vi "Control Experiment SM.vi"() -> ()   [LabVIEW 2016, in "Control Experiment SM.lvclass"]
doc: "Use this VI to help configure your experiment.\n1. Choose Pickering or Not Pickering\n2. Configure the Electrode control to show which electrode is connected to which lockin\n3. Choose a Label for each electrode to configure Krohn Hite amplifier automatically\n4. Easily set all Krohn Hite channels to be \"all ground\" or \"all differential\" mode\n5. Fill out information about you and your device in the lower left corner\n6. When you are finished, or when you want to update the amplifiers, click the \"CREATE OUTPUT\" button located in upper right. Clicking this button will set the amplifiers, Pickering switch (if you have one), and write information to a functional global variable that you can easily read from elsewhere in your program"
uses:
  Control Experiment SM.lvclass
  Typedefs/Instrument--enum.ctl
  <userlib>/LevyLab/Krohn Hite 7008/typedefs/Shunt-Enum.ctl
  <userlib>/LevyLab/Krohn Hite 7008/Instrument.KH7008.lvclass
  <userlib>/LevyLab/Levylab Instruments/SMOs/Configuration/Configuration.lvclass
  <userlib>/LevyLab/Lockin-Multichannel/Instrument.Lockin/Instrument.Lockin.lvclass
  <userlib>/LevyLab/Levylab Instruments/Instrument Types/Cryostat/Instrument.Cryostat.lvclass
  <userlib>/LevyLab/Levylab Instruments/Instrument Types/CBridge/Instrument.CBridge.lvclass
  <userlib>/LevyLab/Levylab Instruments/Instrument Types/Optical Delay Line/Instrument.OpticalDelayLine.lvclass
  <userlib>/LevyLab/Levylab Instruments/Instrument Types/Strain/Instrument.Strain.lvclass
  <userlib>/LevyLab/Levylab Instruments/Instrument Types/VNA/Instrument.VNA.lvclass
  <userlib>/LevyLab/Levylab Instruments/Instrument Types/VSource/Instrument.VSource.lvclass
  Typedefs/KH Mode-enum.ctl
  <userlib>/LevyLab/Krohn Hite 7008/typedefs/Input Configuration-Enum.ctl
  <userlib>/LevyLab/Krohn Hite 7008/typedefs/Gain-Enum.ctl
  <userlib>/LevyLab/Krohn Hite 7008/typedefs/SetAll-Array.ctl
  <userlib>/LevyLab/Krohn Hite 7008/typedefs/SetAll-Cluster.ctl
  <userlib>/LevyLab/Krohn Hite 7008/typedefs/Channel-Enum.ctl
  <userlib>/LevyLab/Krohn Hite 7008/typedefs/Filter-Enum.ctl
  <userlib>/LevyLab/Krohn Hite 7008/typedefs/Coupling-Enum.ctl
  <vilib>/addons/_JKI.lib/REST Client/classes/REST Client/HTTP Header.ctl
  Typedefs/UI Controls --cluster.ctl
  <userlib>/LevyLab/Levylab Instruments/SMOs/Logger.PGSQL/Logger.PGSQL.lvclass
  C:/Program Files (x86)/National Instruments/LabVIEW 2016/vi.lib/JKI/JKI SMO/SMO/SMO.lvclass
  Control Experiment SM.lvclass/Control Experiment SM.ctl
  <vilib>/Utility/sysdir.llb/System Directory Type.ctl
  <userlib>/_MGI/File/MGI Create Directory Chain Behavior Enum.ctl
  Typedefs/Control Experiment JSON--cluster.ctl
  <userlib>/LevyLab/Krohn Hite 7008/Instrument.KH7008.lvclass/Instrument.KH7008.ctl
  <userlib>/_OpenG.lib/file/file.llb/File Exists - Scalar__ogtk.vi
  <vilib>/Platform/browser.llb/Open URL in Default Browser (string).vi
  <userlib>/_OpenG.lib/array/array.llb/Remove Duplicates from 1D Array (Variant)__ogtk.vi
  <vilib>/addons/_JKI.lib/Serialization/JSON/JKI JSON Serialization.lvlib
  <vilib>/addons/_JKI.lib/REST Client/classes/REST Client/REST Client.lvclass
  <vilib>/JKI/JKI SMO/SMO/SMO.lvclass
panel:
  in  "I'm Finished Taking Data!":bool
  out "Values have changed":bool
  in  "Create Output":bool
  in  "OK":bool
  out "Control Experiment":refnum<class "Control Experiment SM.lvclass">
  in  "C.E.":refnum<class "Control Experiment SM.lvclass">
  in  "Tab Control":T1(tab)
  in  "DC Coupled":bool=TRUE
  in  "Bandwidth Filter":bool=TRUE
  in  "#AO":u32=8
  in  "Gain":dbl[](array[numeric])=[1.0, 1.0, 1.0, 1.0, 1.0, 1.0, 1.0, 1.0]
  in  "KH":T5={"KH #"=[0, 1, 2, 3, 4, 5, 6, 7], "KH Configuration"=[enum."Differential", enum."Differential", enum."SE+ (-gnd)", enum."SE+ (-gnd)", enum."Ground", enum."Differential", enum."Ground", enum."Differential"], "KH Gain"=[enum."1x", enum."1000x", enum."1x", enum."10x", enum."1x", enum."1x", enum."1x", enum."1x"], "KH Shunt Resistor"=[enum."50k Ohms", enum."50k Ohms", enum."Open", enum."Open", enum."Open", enum."50k Ohms", enum."Open", enum."Open"]}
  in  "Lockin":T7={"AI"=[1, 2, 3, 4, 5, 6, 7, 8], "Electrode"=["1", "2", "4", "3", "", "26", "", ""], "Label"=[2, 14, 3, 4, 0, 1, 0, 0], "Electrode Config"=[enum."Current", enum."Gate", enum."Voltage (SE)", enum."Voltage (SE)", enum."Ground", enum."Current", enum."Ground", enum."Voltage (Diff)"]} {"Label" items=["", "I+", "I-", "V1+", "V1-", "V2+", "V2-", "V3+", "V3-", "V4+", "V4-", "dV1", "dV2", "dV3", "Vsg", "Vbg"]}
  in  "#AI":u32=8
  in  "KH All Buttons":T8(radio)
  in  "Defualt Shunt Resistor":T4=enum."50k Ohms"
  in  "Description":string="this is a test"
  in  "Sample (SAXXXX)":string="TEST"
  in  "Device (YYYYMMDD)":string="20200113"
  in  "Instrument":T9
  in  "Username":string="Patrick"
  in  "non KH":T10={"AO"=[], "Electrodes 2"=["27"], "Labels 2"=[1], "unused"=[]} {"Labels 2" items=["", "I+", "I-", "V1+", "V1-", "V2+", "V2-", "V3+", "V3-", "V4+", "V4-", "dV1", "dV2", "dV3", "Vsg", "Vbg"]}
  in  "Strain Cell Address":refnum<visa-resource-name>="GPIB0::INSTR38"
  in  "Capacitance Bridge Address":refnum<visa-resource-name>
  in  "C Bridge?":bool=TRUE
  in  "Strain Cell?":bool=TRUE
  in  "Krohn Hite?":bool=TRUE
  in  "KH Addresses":refnum<visa-resource-name>[](array[refnum])=["COM1"] caption="KH Address[A,B,C,...]"
  in  "Lockin Address":string
  in  "Ring":u16(ring) items=["----Sweep Control----", "Sweep Control.vi", "Continuous B Sweep.vi", "----Transport----", "IV.vi", "IV_Sweep.vi", "Lockin_time.vi", "Lockin_Vsg.vi", "Lockin_sweep.vi", "Lockin_AIWFM_time.vi", "THz_TimeDelay.vi", "Sweep_AIWFM_time.vi"]
  in  "Open VI":bool
  in  "Open Lockin":bool
  in  "Write Pickering Config":bool
  in  "Read Pickering Config":bool
  in  "AWS Credentials":path=path "G:/My Drive/ansom/Data" caption="AWS Credentials (File with AWS access key and secret access key"
  out "Refresh Token Out":string="0/0ccae0b202a2d5ce21e5be9cd72246b8"
  in  "Default Path":path=path "G:/My Drive/ansom/Data" caption="Default Path (Do not add your instrument name here)(Typ. G:\\My Drive\\ansom\\Data)"
  out "Comments":string="Device: \r  Device Name: TEST.20200113\r  Computer: ASTARTES\r  User: Patrick\r  Instrument: AGILENT\r  Description: |\r    this is a test\r\rExperiment: \r  Time: 2020-02-25T09:02:18\r  Description: |\r\rSweep: \r- Loop1: [OFF, 0.000000]\r- Loop2: [OFF, 0.000000]\r- Loop3: [OFF, 0.000000]\r- Loop4: [OFF, 0.000000]\r\rWiring: \r- Electrode 27: Lockin 1, I+, KH1 Channel 1, Differential, 1x, 50k Ohms\r\rLockin: \r  AO: \r  \r  REF: \r  \r  Sampling: \r  - Fs: \r  - N: \r"
  out "Device Folder":path=path "G:/My Drive/ansom/Data/AGILENT/TEST.20200113" caption="(\\base path\\project\\device\\ )"
  out "JSON String":string="{\r\n    \"Device\":{\r\n        \"Device\":\"TEST.20200113\",\r\n        \"User\":\"Patrick\",\r\n        \"Time\":\"2020-02-25T09:02:24\",\r\n        \"Computer Name\":\"ASTARTES\"\r\n    },\r\n    \"Wiring\":{\r\n        \"Lockin Ch\":[\r\n            1,\r\n            2,\r\n            3,\r\n            4,\r\n            5,\r\n            6,\r\n            7,\r\n            8\r\n        ],\r\n        \"KH Electrodes\":[\r\n            \"27\"\r\n        ],\r\n        \"KH Labels\":[\r\n            \"I+\"\r\n        ],\r\n        \"Other Electrodes\":[\r\n            \"27\"\r\n        ],\r\n        \"Other Labels\":[\r\n            \"I+\"\r\n        ]\r\n    }\r\n}"
  in  "Labels Strings":string[](array[string])=["", "I+", "I-", "V1+", "V1-", "V2+", "V2-", "V3+", "V3-", "V4+", "V4-", "dV1", "dV2", "dV3", "Vsg", "Vbg"]
  out "YAML example":string="description: This is a dummy dataset which mimics smFRET data.\n\nsetup:\n    ## Mandatory fields\n    num_pixels: 2                # using 2 detectors\n    num_spots: 1                 # a single confocal excitation\n    num_spectral_ch: 2           # donor and acceptor detection\n    num_polarization_ch: 1       # no polarization selection\n    num_split_ch: 1              # no beam splitter\n    modulated_excitation: False  # CW excitation, no modulation\n    lifetime: False              # no TCSPC in detection\n\n    ## Optional fields\n    excitation_wavelengths:      # List of excitation wavelenghts\n       - !!float 532e-9\n    excitation_cw:               # List of booleans, True if wavelength is CW\n       - True\n    detection_wavelengths:       # Nominal center wavelength for each for detection ch\n       - !!float 580e-9\n       - !!float 640e-9\n\nsample:\n  sample_name: describe the sample here\n  buffer_name: describe the buffer here\n  dye_names: 'Cy3B, ATTO647N'   # Comma separates names of fluorophores\n\nidentity:\n    author: Author Name\n    author_affiliation: Name of Research Institution\n\nprovenance:\n    filename: 'photon_data.hdf5'\n    software: Acquisition Software Name\n\nphoton_data:\n    timestamps_specs:\n        timestamps_unit: !!float 10e-9  # 10 ns\n    measurement_specs:\n        measurement_type: smFRET\n        detectors_specs:\n            spectral_ch1: [0]  # list of donor's detector IDs\n            spectral_ch2: [1]  # list of acceptor's detector IDs"
  in  "String":string
  # "SANDBOX:"
  # "Sample"
  # "Krohn Hite"
  # "Lockin"
  # "Lockin"
  # "Krohn Hite"
  # "Other"
  # "Device and Project Description"
  # "Hardware Configuration"
  # "Experiment VIs"
  # "Lockin (Local)"
  # "Path Configuration"
  # "Use this VI to help configure your experiment.\n1. Choose Pickering or Not Pickering\n2. Configure the Electrode control to show which electrode is connected to which lockin\n3. Choose a Label for each electrode to configure Krohn Hite amplifier automatically\n4. Easily set all Krohn Hite channels to be \"all ground\" or \"all differential\" mode\n5. Fill out information about you and your device in the lower left corner\n6. When you are finished, or when you want to update the amplifiers, click the \"CREATE OUTPUT\" button located in upper right.\nClicking this button will set the amplifiers, Pickering switch (if you have one), and write information to a functional global variable that you can easily read from elsewhere in your program"
  # "If you want to have new labels for the \"Labels\" field you can type them here"
  # "The magic words are:\nI\nVsg\nVbg\ndV\nV"
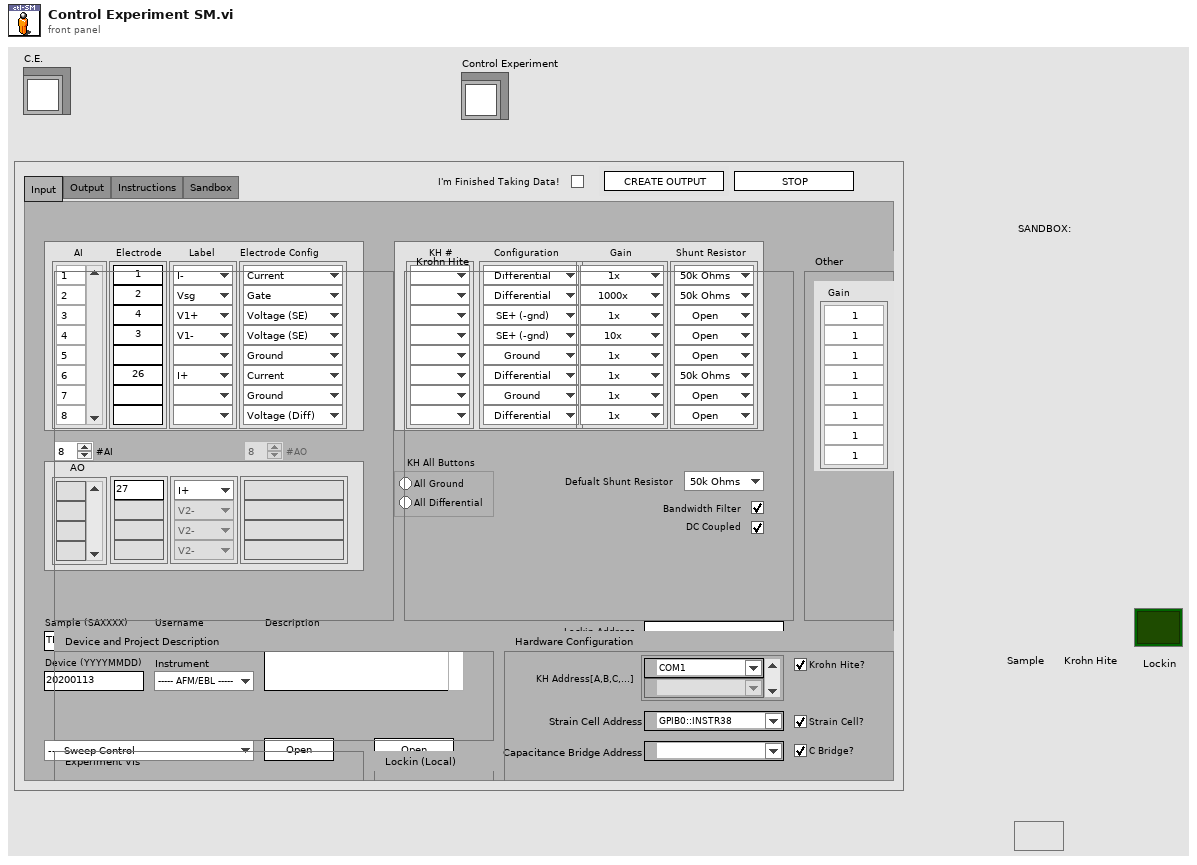
[diagram p1: front panel]
types:
  T1 = enum32{"Input", "Pickering", "Output", "Instructions", "Sandbox"}
  T2 = typedef "Instrument.KH7008.lvclass/Input Configuration-Enum.ctl" = enum16{"Ground", "SE+ (-gnd)", "SE- (+gnd)", "Differential"}
  T3 = typedef "Instrument.KH7008.lvclass/Gain-Enum.ctl" = enum16{"1x", "10x", "100x", "1000x"}
  T4 = typedef "Instrument.KH7008.lvclass/Shunt-Enum.ctl" = enum16{"Open", "50 Ohms", "500 Ohms", "5k Ohms", "50k Ohms", "10M Ohm"}
  T5 = cluster{"KH #":u16[], "KH Configuration":T2[], "KH Gain":T3[], "KH Shunt Resistor":T4[]}
  T6 = typedef "Control Experiment SM.lvclass/KH Mode-enum.ctl" = enum16{"Ground", "Current", "Voltage (SE)", "Voltage (Diff)", "Gate"}
  T7 = cluster{"AI":u32[], "Electrode":string[], "Label":u16[], "Electrode Config":T6[]}
  T8 = enum32{"No Selection", "All Ground", "All Differential"}
  T9 = typedef "Control Experiment SM.lvclass/Instrument--enum.ctl" = enum16{"----- AFM/EBL -----", "AGILENT", "CYPHER", "Gemini2", "JEOL", "MFP3D", "----- Cryostat -----", "CF900", "DR200", "MNK", "PPMS 1", "PPMS 2", "PPMS 3", "----- Optics -----", "THz 1", "THz 2"}
  T10 = cluster{"AO":string[], "Electrodes 2":string[], "Labels 2":u16[], "unused":string[]}
  T11 = enum16{"A 1", "A 2", "A 3", "A 4", "A 5", "A 6", "A 7", "A 8", "B 1", "B 2", "B 3", "B 4", "B 5", "B 6", "B 7", "B 8", "none"}
  T12 = enum32{"invalid app kind", "Development System", "Run Time System", "Student Edition", "Embedded LabVIEW", "Evaluation", "Custom"}
  T13 = enum32{"Invalid", "Standard", "Closed", "Hidden", "Minimized", "Maximized"}
  T14 = typedef "MGI Create Directory Chain Behavior Enum.ctl" = enum16{"Auto Detect", "Path Contains a File", "Path Does Not Contain a File"}
  T15 = typedef "Instrument.KH7008.lvclass/SetAll-Cluster.ctl" = cluster{"Channel":T16, "Gain":T3, "Bandwidth Filter":T17, "Shunt Resistor":T4, "Coupling":T18, "Input Config":T2}
  T16 = typedef "Instrument.KH7008.lvclass/Channel-Enum.ctl" = enum16{"Channel 1", "Channel 2", "Channel 3", "Channel 4", "Channel 5", "Channel 6", "Channel 7", "Channel 8"}
  T17 = typedef "Instrument.KH7008.lvclass/Filter-Enum.ctl" = enum16{"OFF", "ON"}
  T18 = typedef "Instrument.KH7008.lvclass/Coupling-Enum.ctl" = enum16{"AC", "DC"}
  T19 = enum16{"GSR", "Research Projects", "Undergrads", "Researchers", "Hardware", "Software", "LevyLab", "Samples", "Manuscripts", "AoT", "WorkStudy"}
  T20 = enum16{"A 1", "A 2", "A 3", "A 4", "A 5", "A 6", "A 7", "A 8", "B 1", "B 2", "B 3", "B 4", "B 5", "B 6", "B 7", "B 8", "none"}[]
  T21 = typedef "Control Experiment SM.lvclass/Experiment Description--cluster.ctl" = cluster{"User":string, "Device":string, "Device Path":path, "Device Description":string, "Experiment Path":path, "Experiment Description":string, "Instrument":T9, "Sweep":cluster{"key":string, "value":variant}[], "Device Description JSON":string, "Experiment Description JSON":string}
  T22 = typedef "Control Experiment SM.lvclass/Wiring Description--cluster.ctl" = cluster{"Lockin Ch":i32[], "KH":cluster{"Electrodes":string[], "Labels":string[]}, "not KH":cluster{"Electrodes":string[], "Labels":string[]}}
  T23 = typedef "Instrument.KH7008.lvclass/SetAll-Array.ctl" = T15[]
  T24 = typedef "Control Experiment SM.lvclass/UI Controls --cluster.ctl" = cluster{"Sample":string, "Device":string, "Username":string, "Description":string, "Default Path":path, "AWS Path":path, "Instrument":T9, "Lockin?":bool, "Lockin Address":string, "Krohn Hite?":bool, "KH Addresses":refnum<visa-resource-name>[], "KH All Buttons":enum32{"No Selection", "All Ground", "All Differential"}, "Strain Cell?":bool, "Strain Cell Address":refnum<visa-resource-name>, "C Bridge?":bool, "Capacitance Bridge Address":refnum<visa-resource-name>, "Lockin":cluster{"AI":u32[], "Electrode":string[], "Label":u16[], "Electrode Config":T6[]}, "KH":cluster{"KH #":enum16{"A 1", "A 2", "A 3", "A 4", "A 5", "A 6", "A 7", "A 8", "B 1", "B 2", "B 3", "B 4", "B 5", "B 6", "B 7", "B 8", "none"}[], "KH Configuration":T2[], "KH Gain":T3[], "KH Shunt Resistor":T4[], "Filter":bool, "DC Coupled":bool}, "non KH":cluster{"Scroll Bar":string[], "Electrodes 2":string[], "Labels 2":u16[], "unused":string[]}, "#AI":u32}
  T25 = typedef "REST Client.lvlib/REST Client.lvclass/HTTP Header.ctl" = cluster{"header":string, "value":string}
  T26 = cluster{"Core":cluster{"Current VI Reference":refnum<vi>, "Close Panel on Exit?":bool}, "C.E.":refnum<class "Control Experiment SM.lvclass">, "Experiment":T21, "Wiring Configuration":T22, "Channel Settings":cluster{"Channel Setting":T23}[], "KH All Buttons":enum32{"No Selection", "All Ground", "All Differential"}, "Lockin":cluster{"AI":u32[], "Electrode":string[], "Label":u16[], "Electrode Config":T6[]}, "KH":cluster{"KH #":u16[], "KH Configuration":T2[], "KH Gain":T3[], "KH Shunt Resistor":T4[]}, "non KH":cluster{"AO":string[], "Electrodes 2":string[], "Labels 2":u16[], "unused":string[]}, "UI":T24, "Asana":cluster{"Authentication Info":cluster{"Client ID":string, "Client Secret":string, "Redirect URI":string, "Token Endpoint":string, "Scope":string}, "Authentication Header":T25[], "Refresh Token":string, "Time Stamp":timestamp}, "Logger":refnum<class "Logger.PGSQL.lvclass">, "Config":refnum<class "Configuration.lvclass">, "VI paths":path[]}
  T27 = cluster{"Authentication Info":cluster{"Client ID":string, "Client Secret":string, "Redirect URI":string, "Token Endpoint":string, "Scope":string}, "Authentication Header":T25[], "Refresh Token":string, "Time Stamp":timestamp}
  T28 = cluster{"Current VI Reference":refnum<vi>, "Close Panel on Exit?":bool}
  T29 = typedef "System Directory Type.ctl" = i32
  T30 = cluster{"Scroll Bar":string[], "Electrodes 2":string[], "Labels 2":u16[], "unused":string[]}
  T31 = typedef "Control Experiment SM.lvclass/Control Experiment JSON--cluster.ctl" = cluster{"Device":cluster{"Device":string, "User":string, "Time":string, "Computer Name":string}, "Wiring":cluster{"Lockin Ch":u32[], "KH Electrodes":string[], "KH Labels":string[], "Other Electrodes":string[], "Other Labels":string[]}}
  T32 = cluster{"Client ID":string, "Client Secret":string, "Redirect URI":string, "Token Endpoint":string, "Scope":string}
  T33 = cluster{"gid":string, "name":string, "resource_type":string}[]
  T34 = cluster{"id":i64, "gid":string, "resource_type":string, "name":string}[]
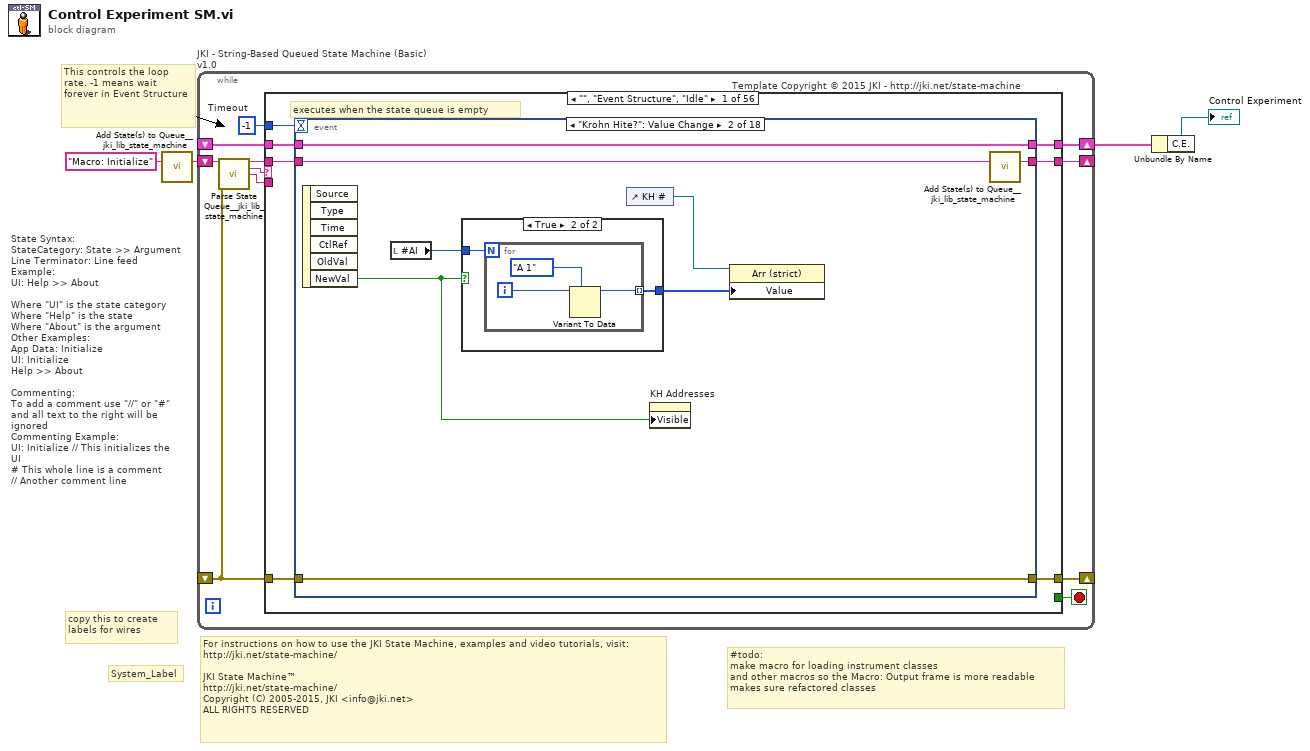
[diagram p0: block diagram]
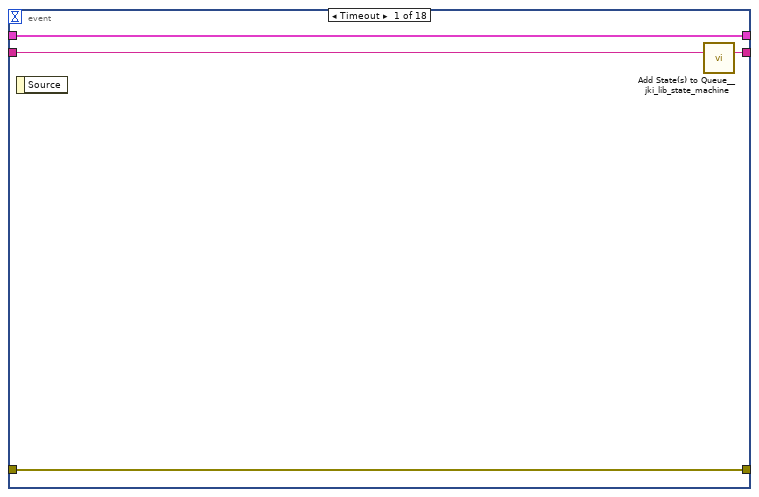
[diagram p2: hidden frame]
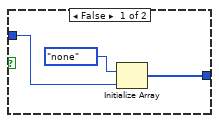
[diagram p3: hidden frame]
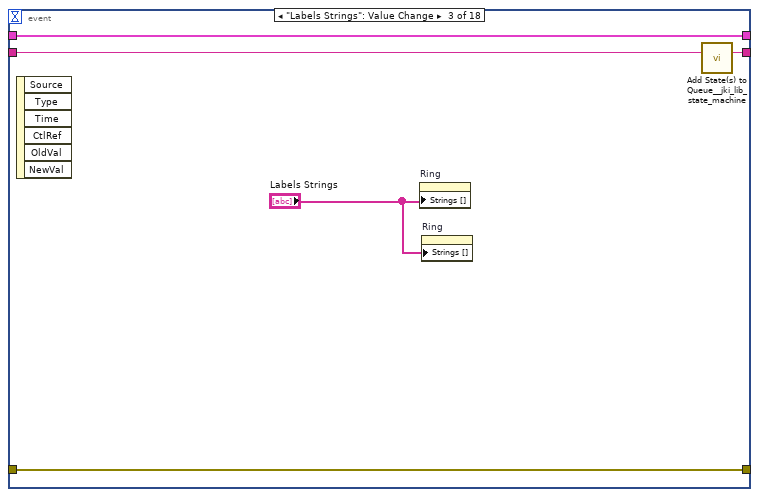
[diagram p4: hidden frame]
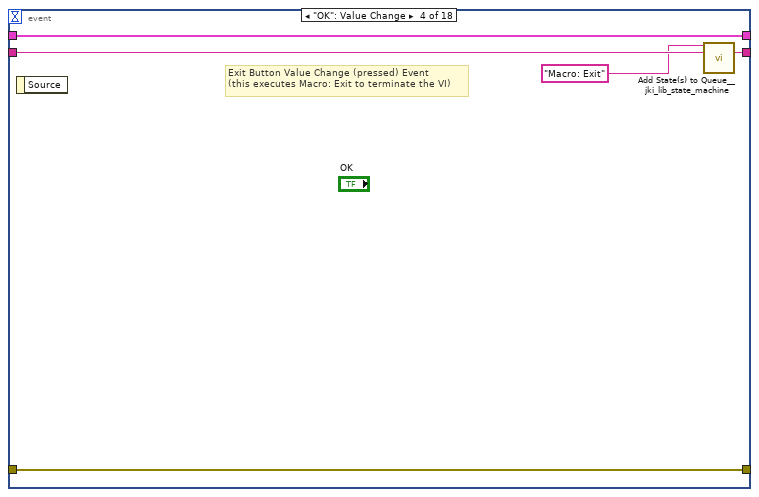
[diagram p5: hidden frame]
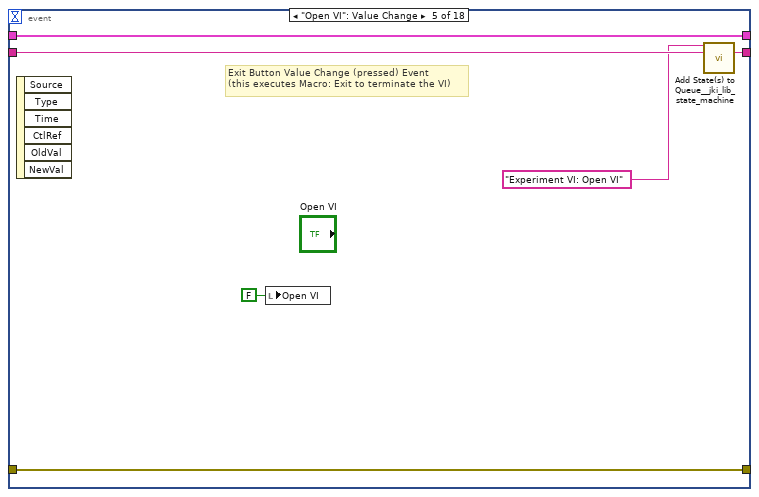
[diagram p6: hidden frame]
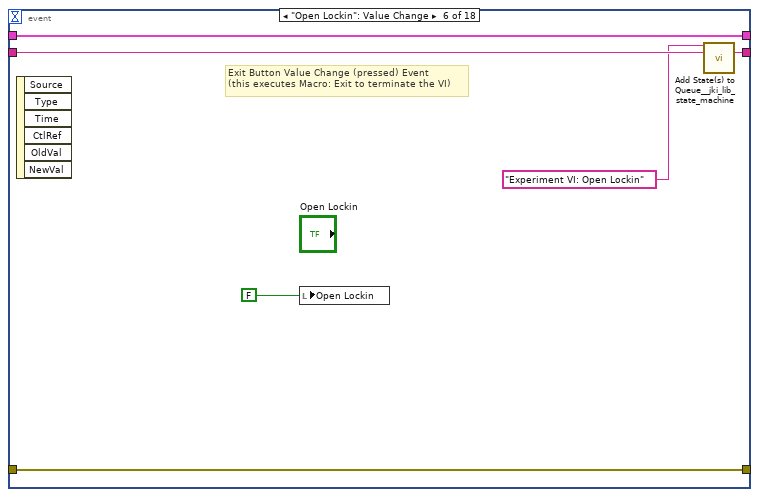
[diagram p7: hidden frame]
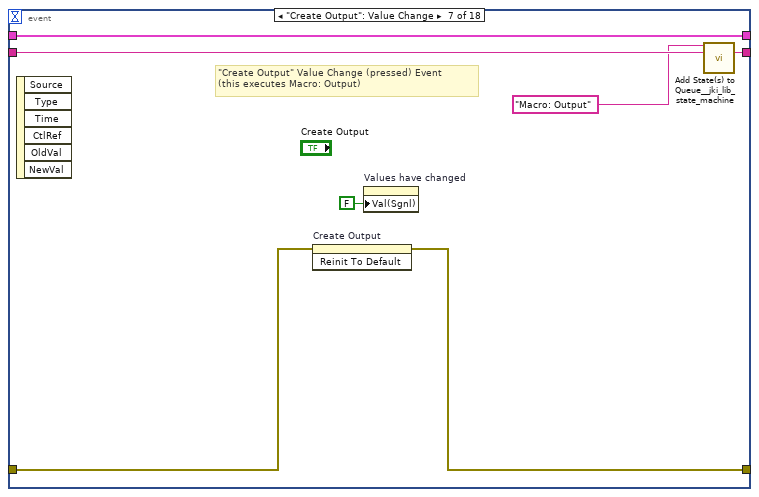
[diagram p8: hidden frame]
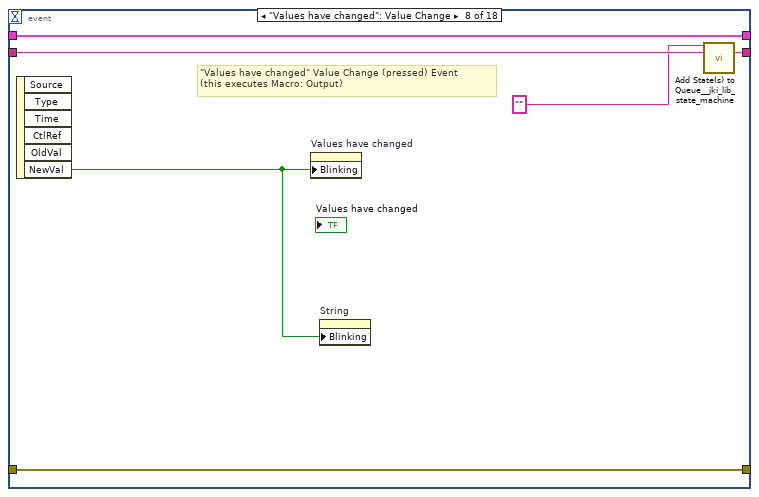
[diagram p9: hidden frame]
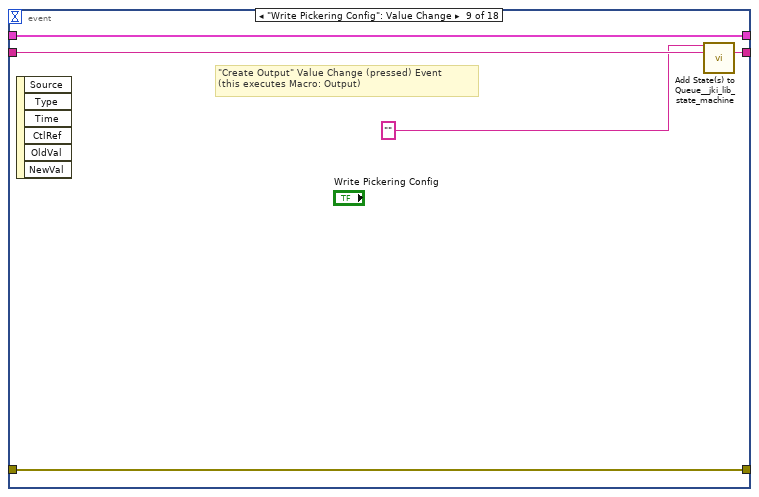
[diagram p10: hidden frame]
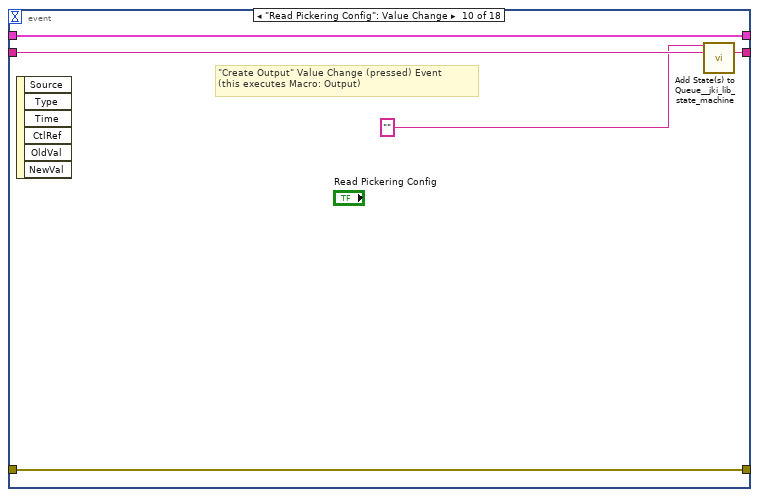
[diagram p11: hidden frame]
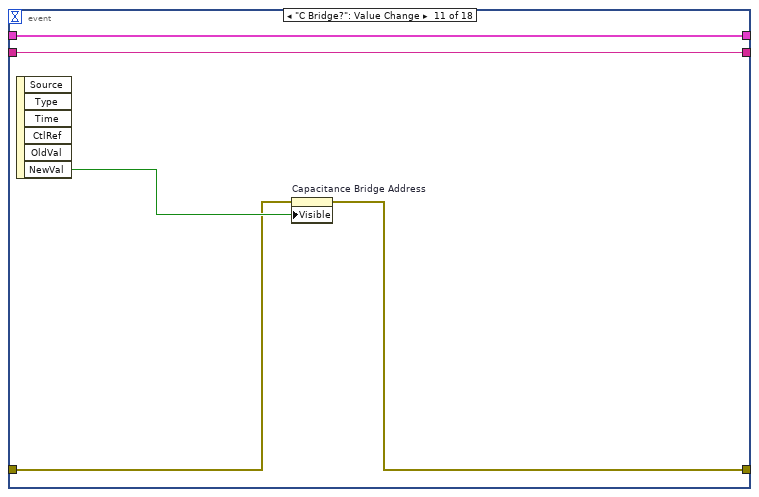
[diagram p12: hidden frame]
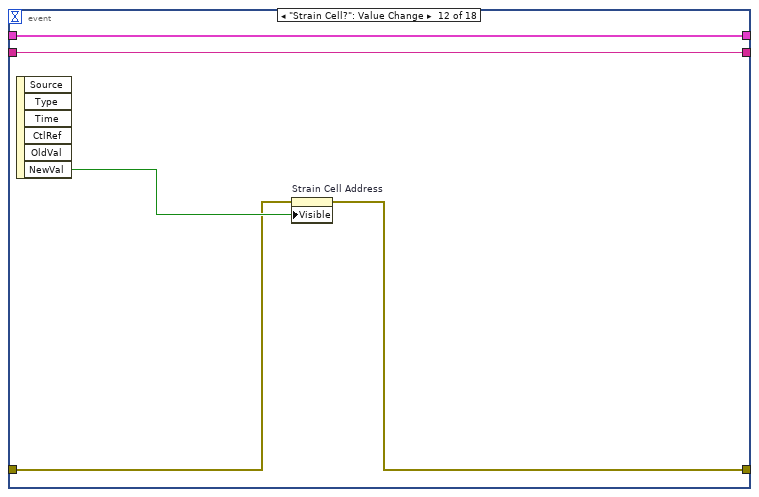
[diagram p13: hidden frame]
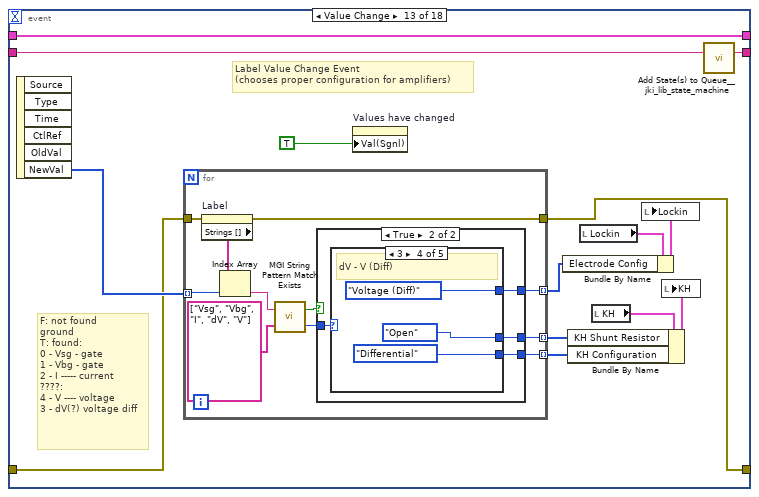
[diagram p14: hidden frame]
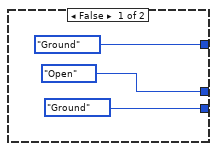
[diagram p15: hidden frame]
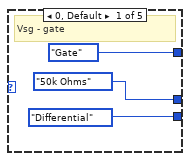
[diagram p16: hidden frame]
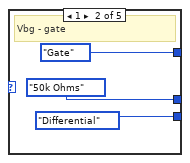
[diagram p17: hidden frame]
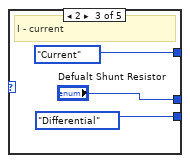
[diagram p18: hidden frame]
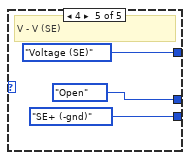
[diagram p19: hidden frame]
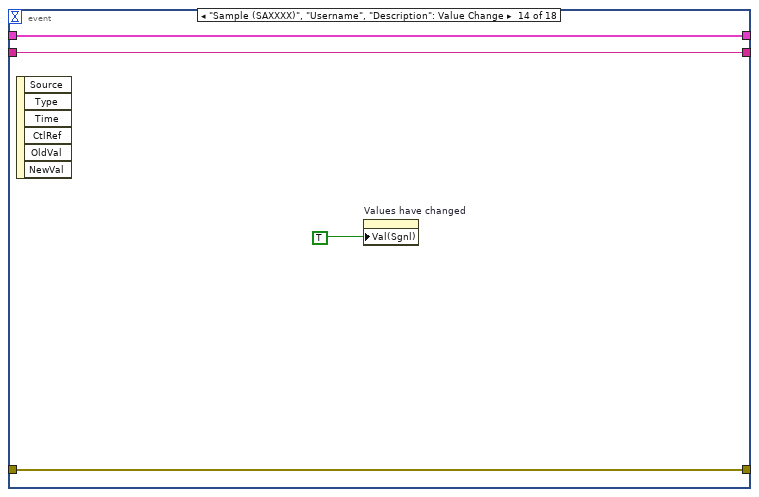
[diagram p20: hidden frame]
diagram:
  # "#todo:\nmake macro for loading instrument classes\nand other macros so the Macro: Output frame is more readable\nmakes sure refactored classes"
  # "For instructions on how to use the JKI State Machine, examples and video tutorials, visit:\nhttp://jki.net/state-machine/\n\nJKI State Machine™\nhttp://jki.net/state-machine/\nCopyright (C) 2005-2015, JKI <info@jki.net>\nALL RIGHTS RESERVED"
  # "State Syntax:\nStateCategory: State >> Argument\nLine Terminator: Line feed\nExample:\nUI: Help >> About\n\nWhere \"UI\" is the state category\nWhere \"Help\" is the state\nWhere \"About\" is the argument\nOther Examples:\nApp Data: Initialize\nUI: Initialize\nHelp >> About\n\nCommenting:\nTo add a comment use \"//\" or \"#\" and all text to the right will be ignored\nCommenting Example:\nUI: Initialize // This initializes the UI\n# This whole line is a comment\n// Another comment line"
  # "copy this to create labels for wires"
  # "This controls the loop rate. -1 means wait forever in Event Structure"
  # "System_Label"
  n1 = call <vilib>:"Add State(s) to Queue__jki_lib_state_machine.vi"("State(s) in (\"\")"="Macro: Initialize") -> ("States Out"=w4:string)  [unwired: 14 in]
  n2 = while "JKI - String-Based Queued State Machine (Basic) v1.0" {
    shift-right: [w8] -> w2
    shift-left: _ -> [w7]
    shift-right: [w11] -> _
    shift-left: _ -> [w5]
    shift-right: [w10] -> _
    shift-left: w4 -> [w12]
    stop <- w9 stop-if-true
    w6 = -1  # Timeout
    # "Template Copyright © 2015 JKI - http://jki.net/state-machine"
    n3 = call <vilib>:"Parse State Queue__jki_lib_state_machine.vi"("State Queue"=w12, "Error In (no error)"=w5) -> ("Remaining States"=w14:string, "Current State"=w15:string, "Arguments"=w13:string)  [unwired: 11 in]
    n4 = case shown="\"\", \"Event Structure\", \"Idle\"" w15 {
      selector: w15 -> [_ _ w189 _ _ _ _ _ _ _ _ _ _ _ _ _ _ _ _ _ _ _ _ _ _ _ _ _ _ _ _ _ _ _ _ _ _ _ _ _ _ _ _ _ _ _ _ _ _ _ _ _ _ _ _ _]
      tunnel: w14 -> [w22 w188 w193 w211 w217 w222 w226 w246 w266 w304 w312 w316 w336 w367 w373 w384 w410 w425 w438 w442 w447 w458 w465 w478 w483 w488 w492 w504 w520 w546 w560 w576 w593 w600 w631 w635 w653 w686 w773 w788 w796 w807 w824 w839 w843 w851 w869 w900 w916 w937 w951 w956 w960 w970 w988 w992]
      tunnel: w13 -> [_ _ _ _ _ _ _ _ _ _ _ _ _ _ w368 w378 _ _ _ _ _ _ _ _ _ _ _ _ _ _ _ _ _ _ _ _ _ _ _ _ _ _ _ _ _ _ _ _ _ _ _ _ _ _ _ _]
      tunnel: w7 -> [w20 w185 w191 w202 w214 w220 w223 _ w262 w283 w307 w313 w324 w340 w371 w380 w407 w422 w436 w439 w444 w455 w463 w475 w480 w485 w489 w500 w516 w543 w558 w572 w591 w598 w603 w632 w651 w678 w764 w785 w794 w800 w820 w831 w840 w845 w853 w885 w913 w924 w949 w954 w957 w962 w986 w989]
      tunnel: [w19 w186 w195 w208 errorcluster {"status"=FALSE, "code"=0, "source"=""} ("error out") w219 w224 w243 w257 w284 w310 w314 w325 w365 w369 w381 w408 w423 w426 w440 w445 w456 w461 w476 w481 w486 w490 w502 w518 w530 w551 w569 w581 w596 w604 w633 w637 w677 w770 w786 w790 w804 w818 w825 w841 w849 w862 w882 w914 w935 w944 w952 w958 w963 w974 w990] -> w11
      tunnel: w5 -> [w18 w186 w194 w208 w213 w219 w224 w243 w263 w285 w308 w314 w334 w365 w370 w382 w408 w423 w433 w440 w445 w456 w461 w476 w481 w486 w490 w502 w518 w533 w552 w569 w582 w594 w619 w633 w647 w677 w759 w786 w789 w805 w821 w832 w841 w849 w852 w898 w914 w935 w945 w953 w958 w964 w976 w990]
      tunnel: [w21 w187 w192 w210 w216 w221 w225 w245 w265 w303 w311 w315 w335 w366 w372 w383 w409 w424 w437 w441 w446 w457 w464 w477 w482 w487 w491 w503 w519 w545 w559 w575 w592 w599 w630 w634 w652 w685 w772 w787 w795 w806 w823 w838 w842 w850 w868 w899 w915 w936 w950 w955 w959 w969 w987 w991] -> w10
      tunnel: [_ _ _ _ _ TRUE _ _ _ _ _ _ _ _ _ _ _ _ _ _ _ _ _ _ _ _ _ _ _ _ _ _ _ _ _ _ _ _ _ _ _ _ _ _ _ _ _ _ _ _ _ _ _ _ _ _] -> w9
      tunnel: [w17 w185 w191 w209 w214 w220 w223 w244 w261 w274 w307 w313 w324 w340 w371 w380 w407 w422 w436 w439 w444 w455 w463 w475 w480 w485 w489 w501 w517 w544 w557 w571 w590 w598 w602 w632 w650 w684 w771 w785 w793 w799 w819 w837 w840 w844 w863 w885 w913 w923 w949 w954 w957 w961 w986 w989] -> w8
      tunnel: w6 -> [w16 _ _ _ _ _ _ _ _ _ _ _ _ _ _ _ _ _ _ _ _ _ _ _ _ _ _ _ _ _ _ _ _ _ _ _ _ _ _ _ _ _ _ _ _ _ _ _ _ _ _ _ _ _ _ _]
      frame "", "Event Structure", "Idle" {
        # "executes when the state queue is empty"
        n5 = event shown="[1] \"Krohn Hite?\": Value Change" {
          selector: _ -> [_ _ _ _ _ _ _ _ _ _ _ _ _ _ _ _ _ _]
          dyn-events: _ -> [_ _ _ _ _ _ _ _ _ _ _ _ _ _ _ _ _ _]
          timeout: w16 -> [_ _ _ _ _ _ _ _ _ _ _ _ _ _ _ _ _ _]
          tunnel: w22 -> [w26 w34 w45 w52 w58 w64 w71 w77 w82 w87 w89 w94 w111 w146 w151 w166 w178 w184]
          tunnel: [w25 w33 w47 w51 w57 w63 w70 w76 w81 w86 w89 w94 w110 w146 w150 w165 w177 w183] -> w21
          tunnel: w20 -> [w23 w31 w46 w49 w55 w61 w69 w75 w80 w85 w88 w93 w109 w147 w152 w164 w175 w181]
          tunnel: [w24 w32 w44 w50 w56 w62 w66 w73 w78 w83 w90 w95 w98 w148 w153 w167 w176 w182] -> w19
          tunnel: w18 -> [w24 w32 w44 w50 w56 w62 w67 w73 w78 w83 w91 w96 w107 w148 w153 w167 w176 w182]
          tunnel: [w23 w31 w46 w49 w55 w61 w69 w75 w80 w85 w88 w93 w109 w147 w152 w164 w175 w181] -> w17
          event Timeout {
            n6 = event-data() -> ()  [unwired: 1 in, 1 out]
            n7 = call <vilib>:"Add State(s) to Queue__jki_lib_state_machine.vi"("State(s) in (\"\")"=w26) -> ("States Out"=w25:string)  [unwired: 14 in]
          }
          event "Krohn Hite?": Value Change {
            n8 = event-data() -> ("NewVal"=w27:bool)  [unwired: 1 in, 5 out]
            n9 = local read "#AI"() -> (w28:u32)
            n10 = case shown="True" w27 {
              tunnel: [w37 w38] -> w29
              tunnel: w28 -> [w36 w39]
              frame False {
                n11 = Initialize Array(T11."none" ("Enum"), w36) -> (w37:T20)
              }
              frame True {
                n12 = for {
                  N: w39 -> [_]
                  tunnel: [w40] -> w38 mode=indexing
                  i -> [w41]
                  n13 = Variant To Data(type=T11."A 1" ("Enum"), Variant=w41) -> (data=w40:T11)  [unwired: 1 in, 1 out]
                }
              }
            }
            n14 = control-ref of="KH #"() -> (w30:refnum<vi>)
            n15 = property on="KH Addresses" class="Arr (strict)"("Visible"=w27) -> ()  [unwired: 2 in, 2 out]
            n16 = property class="Arr (strict)"(reference=w30, "Value"=w29) -> ()  [unwired: 1 in, 2 out]
            n17 = call <vilib>:"Add State(s) to Queue__jki_lib_state_machine.vi"("State(s) in (\"\")"=w34) -> ("States Out"=w33:string)  [unwired: 14 in]
          }
          event "Labels Strings": Value Change {
            n18 = event-data() -> ()  [unwired: 1 in, 6 out]
            n19 = property on="Ring" class="Ring (strict)"("Strings []"="Labels Strings") -> ()  [unwired: 2 in, 2 out]
            n20 = property on="Ring" class="Ring (strict)"("Strings []"="Labels Strings") -> ()  [unwired: 2 in, 2 out]
            n21 = call <vilib>:"Add State(s) to Queue__jki_lib_state_machine.vi"("State(s) in (\"\")"=w45) -> ("States Out"=w47:string)  [unwired: 14 in]
          }
          event "OK": Value Change {
            # "Exit Button Value Change (pressed) Event\n(this executes Macro: Exit to terminate the VI)"
            n22 = event-data() -> ()  [unwired: 1 in, 1 out]
            n23 = call <vilib>:"Add State(s) to Queue__jki_lib_state_machine.vi"("State(s) in Front (\"\")"="Macro: Exit", "State(s) in (\"\")"=w52) -> ("States Out"=w51:string)  [unwired: 13 in]
          }
          event "Open VI": Value Change {
            # "Exit Button Value Change (pressed) Event\n(this executes Macro: Exit to terminate the VI)"
            n24 = event-data() -> ()  [unwired: 1 in, 6 out]
            n25 = local write "Open VI"(FALSE ("Open VI")) -> ()
            n26 = call <vilib>:"Add State(s) to Queue__jki_lib_state_machine.vi"("State(s) in Front (\"\")"="Experiment VI: Open VI", "State(s) in (\"\")"=w58) -> ("States Out"=w57:string)  [unwired: 13 in]
          }
          event "Open Lockin": Value Change {
            # "Exit Button Value Change (pressed) Event\n(this executes Macro: Exit to terminate the VI)"
            n27 = event-data() -> ()  [unwired: 1 in, 6 out]
            n28 = local write "Open Lockin"(FALSE ("Open VI")) -> ()
            n29 = call <vilib>:"Add State(s) to Queue__jki_lib_state_machine.vi"("State(s) in Front (\"\")"="Experiment VI: Open Lockin", "State(s) in (\"\")"=w64) -> ("States Out"=w63:string)  [unwired: 13 in]
          }
          event "Create Output": Value Change {
            # "\"Create Output\" Value Change (pressed) Event\n(this executes Macro: Output)"
            n30 = event-data() -> ()  [unwired: 1 in, 6 out]
            n31 = invoke on="Create Output" class="Bool" method="Reinit To Default"(error in=w67) -> (error out=w66:errorcluster)  [unwired: 2 in, 2 out]
            n32 = property on="Values have changed" class="Bool (strict)"("Val(Sgnl)"=FALSE ("Value (Signaling)")) -> ()  [unwired: 2 in, 2 out]
            n33 = call <vilib>:"Add State(s) to Queue__jki_lib_state_machine.vi"("State(s) in Front (\"\")"="Macro: Output", "State(s) in (\"\")"=w71) -> ("States Out"=w70:string)  [unwired: 13 in]
          }
          event "Values have changed": Value Change {
            # "\"Values have changed\" Value Change (pressed) Event\n(this executes Macro: Output)"
            n34 = event-data() -> ("NewVal"=w72:bool)  [unwired: 1 in, 5 out]
            n35 = property on="Values have changed" class="Bool (strict)"("Blinking"=w72) -> ()  [unwired: 2 in, 2 out]
            n36 = property on="String" class="Str"("Blinking"=w72) -> ()  [unwired: 2 in, 2 out]
            n37 = call <vilib>:"Add State(s) to Queue__jki_lib_state_machine.vi"("State(s) in Front (\"\")"="", "State(s) in (\"\")"=w77) -> ("States Out"=w76:string)  [unwired: 13 in]
          }
          event "Write Pickering Config": Value Change {
            # "\"Create Output\" Value Change (pressed) Event\n(this executes Macro: Output)"
            n38 = event-data() -> ()  [unwired: 1 in, 6 out]
            n39 = call <vilib>:"Add State(s) to Queue__jki_lib_state_machine.vi"("State(s) in Front (\"\")"="", "State(s) in (\"\")"=w82) -> ("States Out"=w81:string)  [unwired: 13 in]
          }
          event "Read Pickering Config": Value Change {
            # "\"Create Output\" Value Change (pressed) Event\n(this executes Macro: Output)"
            n40 = event-data() -> ()  [unwired: 1 in, 6 out]
            n41 = call <vilib>:"Add State(s) to Queue__jki_lib_state_machine.vi"("State(s) in Front (\"\")"="", "State(s) in (\"\")"=w87) -> ("States Out"=w86:string)  [unwired: 13 in]
          }
          event "C Bridge?": Value Change {
            n42 = event-data() -> ("NewVal"=w92:bool)  [unwired: 1 in, 5 out]
            n43 = property on="Capacitance Bridge Address" class="VISAName"(error in=w91, "Visible"=w92) -> (error out=w90:errorcluster)  [unwired: 1 in, 1 out]
          }
          event "Strain Cell?": Value Change {
            n44 = event-data() -> ("NewVal"=w97:bool)  [unwired: 1 in, 5 out]
            n45 = property on="Strain Cell Address" class="VISAName"(error in=w96, "Visible"=w97) -> (error out=w95:errorcluster)  [unwired: 1 in, 1 out]
          }
          event "Lockin.Label": Value Change {
            # "F: not found\nground\nT: found:\n0 - Vsg - gate\n1 - Vbg - gate\n2 - I ----- current\n????:\n4 - V ---- voltage\n3 - dV(?) voltage diff"
            # "Label Value Change Event\n(chooses proper configuration for amplifiers)"
            n46 = event-data() -> ("NewVal"=w108:u16[])  [unwired: 1 in, 5 out]
            n47 = for {
              tunnel: w108 -> [w119] mode=indexing
              tunnel: [w121] -> w103 mode=indexing
              tunnel: w107 -> [w118]
              tunnel: [w117] -> w98
              tunnel: [w116] -> w100 mode=indexing
              tunnel: [w112] -> w101 mode=indexing
              n48 = property on="Label" class="Ring (strict)"(error in=w118) -> (error out=w117:errorcluster, "Strings []"=w120:string[])  [unwired: 1 in, 1 out]
              n49 = Index Array(array=w120, index=w119) -> (element=w115:string)
              n50 = call <userlib>:"MGI String Pattern Match Exists.vi"("Patterns to Try"=string[] ["Vsg", "Vbg", "I", "dV", "V"], "String"=w115) -> ("Index of First Pattern Matched"=w122:i32, "Match Found"=w113:bool)
              n51 = case shown="True" w113 {
                tunnel: w122 -> [_ w129]
                tunnel: [KH_Mode-enum."Ground" ("Enum") w128] -> w121
                tunnel: [Shunt-Enum."Open" ("Shunt Resistor") w127] -> w116
                tunnel: [Input_Configuration-Enum."Ground" ("Input Configuation") w126] -> w112
                frame False {
                }
                frame True {
                  n52 = case shown="3" w129 {
                    tunnel: [KH_Mode-enum."Gate" ("Enum") KH_Mode-enum."Gate" ("Enum") KH_Mode-enum."Current" ("Enum") KH_Mode-enum."Voltage (Diff)" ("Enum") KH_Mode-enum."Voltage (SE)" ("Enum")] -> w128
                    tunnel: [Shunt-Enum."50k Ohms" ("Shunt Resistor") Shunt-Enum."50k Ohms" ("Shunt Resistor") "Defualt Shunt Resistor" Shunt-Enum."Open" ("Shunt Resistor") Shunt-Enum."Open" ("Shunt Resistor")] -> w127
                    tunnel: [Input_Configuration-Enum."Differential" ("Input Configuation") Input_Configuration-Enum."Differential" ("Input Configuation") Input_Configuration-Enum."Differential" ("Input Configuation") Input_Configuration-Enum."Differential" ("Input Configuation") Input_Configuration-Enum."SE+ (-gnd)" ("Input Configuation")] -> w126
                    frame 0, Default {
                      # "Vsg - gate"
                    }
                    frame 1 {
                      # "Vbg - gate"
                    }
                    frame 2 {
                      # "I - current"
                    }
                    frame 3 {
                      # "dV - V (Diff)"
                    }
                    frame 4 {
                      # "V - V (SE)"
                    }
                  }
                }
              }
            }
            n53 = property on="Values have changed" class="Bool (strict)"("Val(Sgnl)"=TRUE ("Values have changed")) -> ()  [unwired: 2 in, 2 out]
            n54 = local read "Lockin"() -> (w105:T7)
            n55 = Bundle By Name(cluster=w105, "Electrode Config"=w103) -> (w104:T7)
            n56 = local read "KH"() -> (w102:T5)
            n57 = Bundle By Name(cluster=w102, "KH Shunt Resistor"=w100, "KH Configuration"=w101) -> (w99:T5)
            n58 = local write "Lockin"(w104) -> ()
            n59 = local write "KH"(w99) -> ()
            n60 = call <vilib>:"Add State(s) to Queue__jki_lib_state_machine.vi"("State(s) in (\"\")"=w111) -> ("States Out"=w110:string)  [unwired: 14 in]
          }
          event "KH.KH Shunt Resistor", "KH.KH Gain", "non KH.Electrodes 2", "non KH.Labels 2", "Sample (SAXXXX)", "Username", "Description", "Lockin.Electrode": Value Change {
            n61 = event-data() -> ()  [unwired: 1 in, 6 out]
            n62 = property on="Values have changed" class="Bool (strict)"("Val(Sgnl)"=TRUE ("Values have changed")) -> ()  [unwired: 2 in, 2 out]
          }
          event "Lockin.AI", "non KH.AO": Mouse Move; "Lockin.AI", "non KH.AO": Mouse Wheel {
            n63 = event-data() -> ()  [unwired: 1 in, 5 out]
            n64 = call <vilib>:"Add State(s) to Queue__jki_lib_state_machine.vi"("State(s) in Front (\"\")"="UI: Link Scroll Bars" ("State(s) in Front (\"\")"), "State(s) in (\"\")"=w151) -> ("States Out"=w150:string)  [unwired: 13 in]
          }
          event "#AI": Value Change {
            n65 = event-data() -> ("NewVal"=w160:u32)  [unwired: 1 in, 5 out]
            n66 = for {
              N: w160 -> [_]
              tunnel: [w169] -> w155 mode=indexing
              tunnel: [w168] -> w154 mode=indexing
              i -> [w168]
              n67 = Increment(x=w168) -> (x+1=w169:i32)
            }
            n68 = local read "Lockin"() -> (w163:T7)
            n69 = Bundle By Name(cluster=w163, "AI"=w155) -> (w162:T7)
            n70 = Initialize Array(1.0 ("element"), w160) -> (w158:dbl[])
            n71 = local read "KH"() -> (w157:T5)
            n72 = local write "Lockin"(w162) -> ()
            n73 = Bundle By Name(cluster=w157, "KH #"=w154) -> (w161:T5)
            n74 = local write "Gain"(w158) -> ()
            n75 = local write "KH"(w161) -> ()
            n76 = call <vilib>:"Add State(s) to Queue__jki_lib_state_machine.vi"("State(s) in Front (\"\")"="KH: set KH 0\nKH: set KH 1" ("State(s) in Front (\"\")"), "State(s) in (\"\")"=w166) -> ("States Out"=w165:string)  [unwired: 13 in]
          }
          event "KH Addresses": Value Change {
            n77 = event-data() -> ()  [unwired: 1 in, 6 out]
            n78 = local read "KH"() -> (w170:T5)
            n79 = Unbundle By Name(w170) -> ("KH #"=w172:u16[])
            n80 = Array Subset(array=w172) -> (w171:u16[])  [unwired: 2 in]
            n81 = Bundle By Name(cluster=w170, "KH #"=w171) -> (w173:T5)
            n82 = local write "KH"(w173) -> ()
            n83 = call <vilib>:"Add State(s) to Queue__jki_lib_state_machine.vi"("State(s) in Front (\"\")"="KH: set KH 0\nKH: set KH 1", "State(s) in (\"\")"=w178) -> ("States Out"=w177:string)  [unwired: 13 in]
          }
          event Panel Close? {
            # "Discard the event because we'll close the front panel ourselves in Macro: Exit"
            # "Close Panel button (pressed) Event\n(this executes Macro: Exit to terminate the VI)"
            n84 = event-data() -> ()  [unwired: 1 in, 1 out]
            n85 = event-data("Discard?"=TRUE) -> ()  [unwired: 1 in, 1 out]
            n86 = call <vilib>:"Add State(s) to Queue__jki_lib_state_machine.vi"("State(s) in Front (\"\")"="Macro: Exit", "State(s) in (\"\")"=w184) -> ("States Out"=w183:string)  [unwired: 13 in]
          }
        }
      }
      frame "---------- Core ----------" {
        # "Do not put any code in this frame.\n(it is a separator no-op)"
        n87 = call <vilib>:"Add State(s) to Queue__jki_lib_state_machine.vi"("State(s) in (\"\")"=w188) -> ("States Out"=w187:string)  [unwired: 14 in]
      }
      frame Default {
        w198 = 42 items=["No error", "Argument error", "Memory is full", "Out of zone", "End of file", "File already open", "Generic file I/O error", "File not found", "File permission error", "Disk is full", "Duplicate path", "Too many files open", "System feature not enabled", "Resource file not found", "Cannot add resource", "Resource not found", "Image not found", "Image memory error", "Pen does not exist", "Config type invalid", "Config token not found", "Config parse error", "Config memory error", "Bad external code format", "Bad external code offset", "External code not present", "Null window", "Destroy window error", "Null menu", "Print aborted", "Bad print record", "Print driver error", "Windows error during printing", "Memory error during printing", "Print dialog error", "Generic print error", "Invalid device refnum", "Device not found", "Device parameter error", "Device unit error", "Cannot open device", "Device call aborted", "Generic error", "Cancelled by user", "Object ID too low", "Object ID too high", "Object not in heap", "Unknown heap", "Unknown object (invalid DefProc)", "Unknown object (DefProc not in table)", "Message out of range", "Invalid (null) method", "Unknown message", "Manager call not supported", "Bad address", "Network operation in progress", "Network operation timed out", "Connection is busy", "Network attribute not supported", "Network error", "Address in use", "System out of memory", "Connection aborted", "Connection refused", "Not connected", "Already connected", "Connection closed", "Initialization error (interapplication manager)", "Bad occurrence", "Wait on unbound occurrence handler", "Occurrence queue overflow", "Datalog type conflict", "Unused", "Unrecognized type (interapplication manager)", "Memory corrupt", "Failed to make temporary DLL", "Old CIN version", "Drag socket not found", "Failed to load drop-object", "Failed to register OLE object", "Failed to release OLE object", "Format specifier type mismatch", "Unknown format specifier", "Too few format specifiers", "Too many format specifiers", "Scan failed", "Newer CIN version", "Error converting to variant", "Runtime menu error", "Password tampered", "Variant attribute not found", "Incompatible variant data type", "Event data is not available", "Event Store is not present", "Occurrence is not found", "Event Queue is not created", "Event info is not available", "Refnum passed is NULL", "Error retrieving Class GUID", "Error retrieving CoClass GUID", "Error retrieving TypeLib GUID.", "Bad built application magic bytes.", "Specific driver is different from the specific driver associated with the Logical Name.", "There is no session opened to the class driver.", "Max Error", "MAX - Error with config objects", "MAX - Error loading configuration", "MAX - Group not supported"]
        # "Current State"
        # "Do not delete, rename, or modify this frame.\n(this is used to capture unhandled states and typos)"
        # "Handle mistyped state name (developer tool)"
        n88 = Format Into String(format string="Software Exception: Unhandled State \"%s\"." ("message"), error in=w194, w189) -> (resulting string=w197:string, error out=w196:errorcluster)  [unwired: 1 in]
        n89 = call <vilib>:"Error Cluster From Error Code.vi"("show call chain? (False)"=TRUE, "error in (no error)"=w196, "error message (\"\")"=w197, "error code (0)"=w198) -> ("error out"=w195:errorcluster)  [unwired: 5 in]
        n90 = call <vilib>:"Add State(s) to Queue__jki_lib_state_machine.vi"("State(s) in (\"\")"=w193) -> ("States Out"=w192:string)  [unwired: 14 in]
      }
      frame "Initialize Core Data" {
        # "Do not delete, rename, or modify this frame.\n(this is used to determine panel behavior on exit)"
        # "originally closed?"
        # "exe?"
        # "If panel starts closed or is an EXE, then close it when we exit"
        n91 = property class="VI"() -> ("Front Panel.Open"=w207:bool)  [unwired: 2 in, 2 out]
        n92 = property class="App"() -> ("App.Kind"=w206:T12)  [unwired: 2 in, 2 out]
        n93 = control-ref of="Current VI Reference"() -> (w200:refnum<vi>)
        n94 = Not(x=w207) -> (.not. x?=w204:bool)
        n95 = Equal?(x=w206, y=T12."Run Time System" ("Application:Kind")) -> (x = y?=w203:bool)
        n96 = Or(x=w204, y=w203) -> (x .or. y?=w201:bool)
        n97 = Bundle By Name(cluster=w202, "Core.Current VI Reference"=w200, "Core.Close Panel on Exit?"=w201) -> (w209:T26)
        n98 = call <vilib>:"Add State(s) to Queue__jki_lib_state_machine.vi"("State(s) in (\"\")"=w211) -> ("States Out"=w210:string)  [unwired: 14 in]
      }
      frame "Error Handler" {
        # "Unhandled Error -- Display it"
        # "Handle any errors here.\nYou can also output any states to clean-up after errors occur"
        # "Clear error"
        n99 = call <vilib>:"General Error Handler.vi"("error in (no error)"=w213) -> ()  [unwired: 10 in, 5 out]
        n100 = call <vilib>:"Add State(s) to Queue__jki_lib_state_machine.vi"("State(s) in Front (\"\")"="/* Post Error States", "State(s) in (\"\")"=w217) -> ("States Out"=w216:string)  [unwired: 13 in]
      }
      frame "Exit" {
        # "Do not put any code in this frame.\n(No errors that occur here will be handled.)"
        n101 = call <vilib>:"Add State(s) to Queue__jki_lib_state_machine.vi"("State(s) in (\"\")"=w222) -> ("States Out"=w221:string)  [unwired: 14 in]
      }
      frame "---------- Data ----------" {
        # "Do not put any code in this frame.\n(It is a separator no-op. You can make a copy of this frame to create a new Data frame)"
        n102 = call <vilib>:"Add State(s) to Queue__jki_lib_state_machine.vi"("State(s) in (\"\")"=w226) -> ("States Out"=w225:string)  [unwired: 14 in]
      }
      frame "Data: Initialize" {
        w228 = path[] []  # VI paths
        w229 = refnum<class "Logger.PGSQL.lvclass"> refnum  # Logger
        w230 = T24 {"Sample"="", "Device"="", "Username"="", "Description"="", "Default Path"=path "", "AWS Path"=path "", "Instrument"=enum."----- AFM/EBL -----", "Lockin?"=FALSE, "Lockin Address"="", "Krohn Hite?"=FALSE, "KH Addresses"=[], "KH All Buttons"=enum."No Selection", "Strain Cell?"=FALSE, "Strain Cell Address"="", "C Bridge?"=FALSE, "Capacitance Bridge Address"="", "Lockin"={"AI"=[], "Electrode"=[], "Label"=[], "Electrode Config"=[]}, "KH"={"KH #"=[], "KH Configuration"=[], "KH Gain"=[], "KH Shunt Resistor"=[], "Filter"=FALSE, "DC Coupled"=FALSE}, "non KH"={"Scroll Bar"=[], "Electrodes 2"=[], "Labels 2"=[], "unused"=[]}, "#AI"=8}  # UI
        w236 = refnum<class "Configuration.lvclass"> refnum  # Config
        w239 = T27 {"Authentication Info"={"Client ID"="1150712142949183", "Client Secret"="530770942aed47201cd52aeb331bdd57", "Redirect URI"="https://www.google.com/", "Token Endpoint"="https://app.asana.com/-/oauth_token", "Scope"=""}, "Authentication Header"=[], "Refresh Token"="", "Time Stamp"=timestamp(0 s since 1904-01-01)}  # Asana
        w240 = cluster{"Channel Setting":T23}[] []  # Channel Settings
        w234 = T28 {"Current VI Reference"=refnum, "Close Panel on Exit?"=FALSE}  # Core
        # "Initialize the shift-register data, here.\n(data names are defined by what you wire into the bundle function)"
        n103 = local read "Refresh Token Out"() -> (w238:string)
        n104 = Unbundle By Name("C.E.") -> ("Experiment"=w241:T21, "Wiring Configuration"=w242:T22)
        n105 = Bundle By Name(cluster=w239, "Refresh Token"=w238) -> (w237:T27)
        n106 = Bundle("Core"=w234, "C.E."="C.E.", "Experiment"=w241, "Wiring Configuration"=w242, "Channel Settings"=w240, "KH All Buttons"="KH All Buttons", "Lockin"="Lockin", "KH"="KH", "non KH"="non KH", "UI"=w230, "Asana"=w237, "Logger"=w229, "Config"=w236, "VI paths"=w228) -> (w244:T26)  [unwired: 1 in]
        n107 = call <vilib>:"Add State(s) to Queue__jki_lib_state_machine.vi"("State(s) in (\"\")"=w246) -> ("States Out"=w245:string)  [unwired: 14 in]
      }
      frame "Data: Load Configuration" {
        w252 = T29 3 items=["User Home"=0, "User Desktop"=1, "User Documents"=2, "User Application Data"=3, "User Preferences"=4, "User Temporary"=5, "Public Documents"=6, "Public Application Data"=7, "Public Preferences"=8, "Public Cache"=13, "System Core Libraries"=9, "System Installed Libraries"=10, "Application Files"=11, "Boot Volume Root"=12] ("system directory type")
        n108 = disable-structure shown="Disabled" {
          frame Disabled {
            w270 = T29 7 items=["User Home"=0, "User Desktop"=1, "User Documents"=2, "User Application Data"=3, "User Preferences"=4, "User Temporary"=5, "Public Documents"=6, "Public Application Data"=7, "Public Preferences"=8, "Public Cache"=13, "System Core Libraries"=9, "System Installed Libraries"=10, "Application Files"=11, "Boot Volume Root"=12] ("system directory type")
            n109 = call <vilib>:"Get System Directory.vi"("system directory type"=w270) -> ("system directory"=w267:path)  [unwired: 10 in]
            n110 = Build Path(base path=w267, name or relative path="Levylab") -> (appended path=w269:path)
            n111 = Build Path(base path=w269, name or relative path="Control Experiment") -> ()  [unwired: 1 out]
          }
          frame Enabled {
          }
        }
        n112 = Unbundle By Name(w262) -> ("Config"=w264:refnum<class "Configuration.lvclass">, "UI"=w256:T24)
        n113 = call <vilib>:"Get System Directory.vi"("system directory type"=w252) -> ("system directory"=w251:path)  [unwired: 10 in]
        n114 = Build Path(base path=w251, name or relative path="LevyLab") -> (appended path=w249:path)
        n115 = Build Path(base path=w249, name or relative path="Control Experiment") -> (appended path=w247:path)
        n116 = call <userlib>:"Write Path.vi"("error in (no error)"=w263, "Path"=w247, "Configuration in"=w264) -> ("error out"=w259:errorcluster, "Configuration out"=w260:refnum<class "Configuration.lvclass">)  [unwired: 7 in]
        n117 = call <userlib>:"Read Configuration.vi"("INI Fomatted Cluster Type"=w256, "error in (no error)"=w259, "Configuration in"=w260) -> ("error out"=w258:errorcluster, "Configuration"=w254:variant, "Configuration out"=w255:refnum<class "Configuration.lvclass">)  [unwired: 6 in]
        n118 = Variant To Data(error in=w258, type=w256, Variant=w254) -> (data=w253:T24, error out=w257:errorcluster)
        n119 = Bundle By Name(cluster=w262, "Config"=w255, "UI"=w253) -> (w261:T26)
        n120 = call <vilib>:"Add State(s) to Queue__jki_lib_state_machine.vi"("State(s) in (\"\")"=w266) -> ("States Out"=w265:string)  [unwired: 14 in]
      }
      frame "Data: Save Controls" {
        n121 = local read "Sample (SAXXXX)"() -> (w302:string)
        n122 = local read "Username"() -> (w300:string)
        n123 = local read "Default Path"() -> (w298:path)
        n124 = local read "Strain Cell?"() -> (w292:bool)
        n125 = local read "C Bridge?"() -> (w290:bool)
        n126 = local read "Lockin"() -> (w288:T7)
        n127 = local read "Lockin Address"() -> (w296:string)
        n128 = local read "KH Addresses"() -> (w294:refnum<visa-resource-name>[])
        n129 = local read "KH"() -> (w281:T5)
        n130 = local read "Description"() -> (w299:string)
        n131 = local read "Strain Cell Address"() -> (w291:refnum<visa-resource-name>)
        n132 = local read "Capacitance Bridge Address"() -> (w289:refnum<visa-resource-name>)
        n133 = local read "Instrument"() -> (w297:T9)
        n134 = local read "Device (YYYYMMDD)"() -> (w301:string)
        n135 = Unbundle By Name(w281) -> ("KH #"=w280:u16[], "KH Configuration"=w277:T2[], "KH Gain"=w278:T3[], "KH Shunt Resistor"=w279:T4[])
        n136 = local read "Krohn Hite?"() -> (w295:bool)
        n137 = local read "KH All Buttons"() -> (w293:T8)
        n138 = local read "AWS Credentials"() -> (w273:path)
        n139 = local read "non KH"() -> (w282:T10)
        n140 = local read "#AI"() -> (w272:u32)
        n141 = Bundle By Name(cluster=w283, "UI.Sample"=w302, "UI.Device"=w301, "UI.Username"=w300, "UI.Description"=w299, "UI.Default Path"=w298, "UI.AWS Path"=w273, "UI.Instrument"=w297, "UI.Lockin Address"=w296, "UI.Krohn Hite?"=w295, "UI.KH Addresses"=w294, "UI.KH All Buttons"=w293, "UI.Strain Cell?"=w292, "UI.Strain Cell Address"=w291, "UI.C Bridge?"=w290, "UI.Capacitance Bridge Address"=w289, "UI.Lockin"=w288, "UI.non KH"=w282, "UI.KH.KH #"=w280, "UI.KH.KH Configuration"=w277, "UI.KH.KH Gain"=w278, "UI.KH.KH Shunt Resistor"=w279, "UI.KH.Filter"="Bandwidth Filter", "UI.KH.DC Coupled"="DC Coupled", "UI.#AI"=w272) -> (w274:T26)
        n142 = Unbundle By Name(w274) -> ("Config"=w287:refnum<class "Configuration.lvclass">, "UI"=w286:T24)
        n143 = call <userlib>:"Write Configuration.vi"("error in (no error)"=w285, "Variant"=w286, "Configuration in"=w287) -> ("error out"=w284:errorcluster)  [unwired: 7 in, 1 out]
        n144 = call <vilib>:"Add State(s) to Queue__jki_lib_state_machine.vi"("State(s) in (\"\")"=w304) -> ("States Out"=w303:string)  [unwired: 14 in]
      }
      frame "Data: Cleanup" {
        # "Cleanup any data and references, here.\n(this is called automatically, by the Macro: Exit)"
        n145 = Unbundle By Name(w307) -> ("Core.Current VI Reference"=w306:refnum<vi>, "Logger"=w309:refnum<class "Logger.PGSQL.lvclass">)
        n146 = call <vilib>:"Stop.vi"("error in (no error)"=w308, "SMO"=w309) -> ("error out"=w305:errorcluster)  [unwired: 8 in, 1 out]
        n147 = Close Reference(reference=w306, error in (no error)=w305) -> (error out=w310:errorcluster)
        n148 = call <vilib>:"Add State(s) to Queue__jki_lib_state_machine.vi"("State(s) in (\"\")"=w312) -> ("States Out"=w311:string)  [unwired: 14 in]
      }
      frame "---------- UI ----------" {
        # "Do not put any code in this frame.\n(It is a separator no-op. You can make a copy of this frame to create a new UI frame)"
        n149 = call <vilib>:"Add State(s) to Queue__jki_lib_state_machine.vi"("State(s) in (\"\")"=w316) -> ("States Out"=w315:string)  [unwired: 14 in]
      }
      frame "UI: Initialize" {
        w318 = TRUE ("Visible")
        (unwired) string[] ["", "I+", "I-", "V1+", "V1-", "V2+", "V2-", "V3+", "V3-", "V4+", "V4-", "dV1", "dV2", "dV3", "Vsg", "Vbg"] ("Strings [] 2")
        # "Pickering? = False always"
        # "unused"
        # "Initialize the User Interface, here.\n(this is called automatically, by the Macro: Init)"
        n150 = local read "Labels Strings"() -> (w329:string[])
        n151 = call <userlib>:"Fit VI window to Largest Dec__ogtk.vi"("error in (no error)"=w334) -> ("error out"=w331:errorcluster)  [unwired: 5 in, 1 out]
        n152 = Unbundle By Name(w324) -> ("UI.Krohn Hite?"=w321:bool, "UI.Strain Cell?"=w320:bool, "UI.C Bridge?"=w319:bool)
        n153 = property on="OK" class="Bool (strict)"("Value"=FALSE ("Blinking")) -> ()  [unwired: 2 in, 2 out]
        n154 = property on="Ring" class="Ring (strict)"(error in=w331, "Strings []"=w329) -> (error out=w330:errorcluster)  [unwired: 1 in, 1 out]
        n155 = local write "KH All Buttons"(T8."No Selection" ("KH All Buttons")) -> ()
        n156 = property on="Values have changed" class="Bool (strict)"("Val(Sgnl)"=FALSE ("Blinking")) -> ()  [unwired: 2 in, 2 out]
        n157 = property on="Ring" class="Ring (strict)"(error in=w330, "Strings []"=w329) -> (error out=w332:errorcluster)  [unwired: 1 in, 1 out]
        n158 = property on="Tab Control" class="TabCtl (strict)"("Value"=T1."Input" ("Tab Control")) -> ()  [unwired: 2 in, 2 out]
        n159 = property on="Krohn Hite?" class="Bool (strict)"("Val(Sgnl)"=w321, "Visible"=w318) -> ()  [unwired: 2 in, 2 out]
        n160 = property on="#AI" class="DigNum (strict)"("Val(Sgnl)"="#AI") -> ()  [unwired: 2 in, 2 out]
        n161 = disable-structure shown="Enabled" {
          disable-tunnel: w332 -> [_ w337]
          disable-tunnel: [_ w337] -> w325
          disable-tunnel: FALSE ("Blinking") -> [_ _]
          frame Disabled {
          }
          frame Enabled {
          }
        }
        n162 = property on="Strain Cell?" class="Bool (strict)"("Val(Sgnl)"=w320, "Visible"=w318) -> ()  [unwired: 2 in, 2 out]
        n163 = local read "KH Addresses"() -> (w322:refnum<visa-resource-name>[])
        n164 = property on="C Bridge?" class="Bool (strict)"("Val(Sgnl)"=w319, "Visible"=w318) -> ()  [unwired: 2 in, 2 out]
        n165 = property on="KH Addresses" class="Arr (strict)"("Val(Sgnl)"=w322) -> ()  [unwired: 2 in, 2 out]
        n166 = call <vilib>:"Add State(s) to Queue__jki_lib_state_machine.vi"("State(s) in (\"\")"=w336) -> ("States Out"=w335:string)  [unwired: 14 in]
      }
      frame "UI: Update Controls" {
        # "Do not put any code in this frame.\n(It is a separator no-op. You can make a copy of this frame to create a new Data frame)"
        n167 = Unbundle By Name(w340) -> ("UI.Sample"=w356:string, "UI.Device"=w357:string, "UI.Username"=w358:string, "UI.Description"=w359:string, "UI.Default Path"=w364:path, "UI.AWS Path"=w339:path, "UI.Instrument"=w360:T9, "UI.Lockin Address"=w354:string, "UI.Krohn Hite?"=w363:bool, "UI.KH Addresses"=w355:refnum<visa-resource-name>[], "UI.KH All Buttons"=w351:T8, "UI.Strain Cell?"=w362:bool, "UI.Strain Cell Address"=w352:refnum<visa-resource-name>, "UI.C Bridge?"=w361:bool, "UI.Capacitance Bridge Address"=w353:refnum<visa-resource-name>, "UI.Lockin"=w350:T7, "UI.non KH"=w349:T30, "UI.KH.Filter"=w347:bool, "UI.KH.DC Coupled"=w348:bool, "UI.KH.KH #"=w344:T20, "UI.KH.KH Configuration"=w343:T2[], "UI.KH.KH Gain"=w342:T3[], "UI.KH.KH Shunt Resistor"=w341:T4[], "UI.#AI"=w338:u32)
        n168 = local write "Sample (SAXXXX)"(w356) -> ()
        n169 = local write "Krohn Hite?"(w363) -> ()
        n170 = local write "Bandwidth Filter"(w347) -> ()
        n171 = local write "Strain Cell?"(w362) -> ()
        n172 = local write "C Bridge?"(w361) -> ()
        n173 = local write "Username"(w358) -> ()
        n174 = local write "Lockin"(w350) -> ()
        n175 = local write "Instrument"(w360) -> ()
        n176 = local write "Default Path"(w364) -> ()
        n177 = local write "KH Addresses"(w355) -> ()
        n178 = local write "Strain Cell Address"(w352) -> ()
        n179 = local write "Capacitance Bridge Address"(w353) -> ()
        n180 = local write "DC Coupled"(w348) -> ()
        n181 = local write "non KH"(w349) -> ()
        n182 = local write "Device (YYYYMMDD)"(w357) -> ()
        n183 = local write "#AI"(w338) -> ()
        n184 = local write "AWS Credentials"(w339) -> ()
        n185 = local write "Description"(w359) -> ()
        n186 = local write "Lockin Address"(w354) -> ()
        n187 = local write "KH All Buttons"(w351) -> ()
        n188 = local read "KH"() -> (w346:T5)
        n189 = Bundle By Name(cluster=w346, "KH #"=w344, "KH Configuration"=w343, "KH Gain"=w342, "KH Shunt Resistor"=w341) -> (w345:T5)
        n190 = local write "KH"(w345) -> ()
        n191 = call <vilib>:"Add State(s) to Queue__jki_lib_state_machine.vi"("State(s) in (\"\")"=w367) -> ("States Out"=w366:string)  [unwired: 14 in]
      }
      frame "UI: Cursor Set" {
        # "Argument"
        # "Set and Unset Cursor Busy.\n(Usage: \"UI: Cursor Set >> Busy|Idle\")"
        n192 = case shown="\"Busy\"" w368 {
          tunnel: w370 -> [w375 w377]
          tunnel: [w374 w376] -> w369
          frame "Idle", Default {
            n193 = call <vilib>:"Unset Busy.vi"("error in (no error)"=w375) -> ("error out"=w374:errorcluster)  [unwired: 10 in]
          }
          frame "Busy" {
            n194 = call <vilib>:"Set Busy.vi"("error in (no error)"=w377) -> ("error out"=w376:errorcluster)  [unwired: 9 in, 1 out]
          }
        }
        n195 = call <vilib>:"Add State(s) to Queue__jki_lib_state_machine.vi"("State(s) in (\"\")"=w373) -> ("States Out"=w372:string)  [unwired: 14 in]
      }
      frame "UI: Front Panel State" {
        # "Argument"
        # "Set Front Panel Open or Closed\n(Usage: \"UI: Front Panel State >> Open|Close\")"
        n196 = Unbundle By Name(w380) -> ("Core.Current VI Reference"=w379:refnum<vi>)
        n197 = case shown="\"Open\", Default" w378 {
          tunnel: w382 -> [w388 w401]
          tunnel: [w390 w402] -> w381
          tunnel: w379 -> [w389 w399]
          frame "Open", Default {
            n198 = property class="VI"(reference=w389, error in=w388) -> (reference out=w386:refnum<vi>, error out=w387:errorcluster, "Front Panel.Open"=w385:bool)
            n199 = case shown="True" w385 {
              tunnel: [w393 w396] -> w390
              tunnel: w387 -> [w392 w396]
              tunnel: w386 -> [w391 _]
              frame False {
                n200 = invoke class="VI" method="FP.Open"(reference=w391, error in=w392, "Activate"=TRUE, "State"=T13."Standard") -> (error out=w393:errorcluster)  [unwired: 1 in, 4 out]
              }
              frame True {
              }
            }
          }
          frame "Close" {
            n201 = property class="VI"(reference=w399, error in=w401) -> (reference out=w398:refnum<vi>, error out=w400:errorcluster, "Front Panel.Open"=w397:bool)
            n202 = case shown="True" w397 {
              tunnel: [w403 w406] -> w402
              tunnel: w400 -> [w403 w405]
              tunnel: w398 -> [_ w404]
              frame False {
              }
              frame True {
                n203 = invoke class="VI" method="FP.Close"(reference=w404, error in=w405) -> (error out=w406:errorcluster)  [unwired: 1 in, 2 out]
              }
            }
          }
        }
        n204 = call <vilib>:"Add State(s) to Queue__jki_lib_state_machine.vi"("State(s) in (\"\")"=w384) -> ("States Out"=w383:string)  [unwired: 14 in]
      }
      frame "UI: Buttons" {
        # "Do not put any code in this frame.\n(It is a separator no-op. You can make a copy of this frame to create a new UI frame)"
        n205 = call <vilib>:"Add State(s) to Queue__jki_lib_state_machine.vi"("State(s) in (\"\")"=w410) -> ("States Out"=w409:string)  [unwired: 14 in]
      }
      frame "UI: Link Scroll Bars" {
        # "Do not put any code in this frame.\n(It is a separator no-op. You can make a copy of this frame to create a new UI frame)"
        n206 = control-ref of="AI"() -> (w421:refnum<vi>)
        n207 = control-ref of="Electrode"() -> (w420:refnum<vi>)
        n208 = control-ref of="Label"() -> (w419:refnum<vi>)
        n209 = control-ref of="Electrode Config"() -> (w418:refnum<vi>)
        n210 = control-ref of="KH #"() -> (w417:refnum<vi>)
        n211 = control-ref of="KH Configuration"() -> (w416:refnum<vi>)
        n212 = control-ref of="KH Gain"() -> (w415:refnum<vi>)
        n213 = control-ref of="KH Shunt Resistor"() -> (w414:refnum<vi>)
        n214 = control-ref of="Gain"() -> (w412:refnum<vi>)
        n215 = property class="Arr (strict)"(reference=w421) -> ("Index Values"=w411:u32[])  [unwired: 1 in, 2 out]
        n216 = property class="Arr (strict)"(reference=w420, "Index Values"=w411) -> ()  [unwired: 1 in, 2 out]
        n217 = property class="Arr (strict)"(reference=w419, "Index Values"=w411) -> ()  [unwired: 1 in, 2 out]
        n218 = property class="Arr (strict)"(reference=w418, "Index Values"=w411) -> ()  [unwired: 1 in, 2 out]
        n219 = property class="Arr (strict)"(reference=w417, "Index Values"=w411) -> ()  [unwired: 1 in, 2 out]
        n220 = property class="Arr (strict)"(reference=w416, "Index Values"=w411) -> ()  [unwired: 1 in, 2 out]
        n221 = property class="Arr (strict)"(reference=w415, "Index Values"=w411) -> ()  [unwired: 1 in, 2 out]
        n222 = property class="Arr (strict)"(reference=w414, "Index Values"=w411) -> ()  [unwired: 1 in, 2 out]
        n223 = property class="Arr (strict)"(reference=w412, "Index Values"=w411) -> ()  [unwired: 1 in, 2 out]
        n224 = property on="AO" class="Arr (strict)"() -> ("Index Values"=w413:u32[])  [unwired: 2 in, 2 out]
        n225 = property on="Labels 2" class="Arr (strict)"("Index Values"=w413) -> ()  [unwired: 2 in, 2 out]
        n226 = property on="unused" class="Arr (strict)"("Index Values"=w413) -> ()  [unwired: 2 in, 2 out]
        n227 = property on="Electrodes 2" class="Arr (strict)"("Index Values"=w413) -> ()  [unwired: 2 in, 2 out]
        n228 = call <vilib>:"Add State(s) to Queue__jki_lib_state_machine.vi"("State(s) in (\"\")"=w425) -> ("States Out"=w424:string)  [unwired: 14 in]
      }
      frame "UI: SR Disable" {
        # "Do not put any code in this frame.\n(It is a separator no-op. You can make a copy of this frame to create a new UI frame)"
        n229 = local read "KH Addresses"() -> (w435:refnum<visa-resource-name>[])
        n230 = control-ref of="Shunt Resistor"() -> (w431:refnum<vi>)
        n231 = Index Array(array=w435) -> (element=w434:refnum<visa-resource-name>)  [unwired: 1 in]
        n232 = call <userlib>:"Shunt - Check 500 or 10M.vi"("error in (no error)"=w433, "VISA Refnum in"=w434) -> ("error out"=w432:errorcluster, "SR"=w428:enum16{"500", "10M"})  [unwired: 7 in, 1 out]
        n233 = call <vilib>:"Clear Errors.vi"("error in (no error)"=w432) -> ("error out"=w430:errorcluster)  [unwired: 5 in, 1 out]
        n234 = call <userlib>:"Shunt - 500 or 10M Control Disable.vi"("error in"=w430, "SR"=w428, "reference"=w431) -> ("error out"=w427:errorcluster)  [unwired: 8 in]
        n235 = control-ref of="Defualt Shunt Resistor"() -> (w429:refnum<vi>)
        n236 = call <userlib>:"Shunt - 500 or 10M Control Disable.vi"("error in"=w427, "SR"=w428, "reference"=w429) -> ("error out"=w426:errorcluster)  [unwired: 8 in]
        n237 = call <vilib>:"Add State(s) to Queue__jki_lib_state_machine.vi"("State(s) in (\"\")"=w438) -> ("States Out"=w437:string)  [unwired: 14 in]
      }
      frame "---------- Macro ----------" {
        # "Do not put any code in this frame.\n(It is a separator no-op. You can make a copy of this frame to create a new Macro frame)"
        n238 = call <vilib>:"Add State(s) to Queue__jki_lib_state_machine.vi"("State(s) in (\"\")"=w442) -> ("States Out"=w441:string)  [unwired: 14 in]
      }
      frame "Macro: Initialize" {
        # "Initialization Macro\n(This is called once, when the VI starts)"
        n239 = call <vilib>:"Add State(s) to Queue__jki_lib_state_machine.vi"("State(s) in Front (\"\")"="Data: Initialize\nInitialize Core Data\nData: Load Configuration\nUI: Update Controls\nUI: Initialize\nUI: Front Panel State >> Open\nUI: SR Disable\nExperiment VI: Populate VI Ring\n//Asana: Initialize Authentication Info\n//Macro: Asana\nPGSQL: Start Logger", "State(s) in (\"\")"=w447) -> ("States Out"=w446:string)  [unwired: 13 in]
      }
      frame "Macro: Exit" {
        # "Exit Macro\n(This is called once, when the VI exits)"
        n240 = Unbundle By Name(w455) -> ("Core.Close Panel on Exit?"=w454:bool)
        n241 = property on="OK" class="Bool (strict)"("Value"=FALSE ("Blinking")) -> ()  [unwired: 2 in, 2 out]
        n242 = Select(t="UI: Front Panel State >> Close", s=w454, f="") -> (s? t:f=w451:string)
        n243 = call <vilib>:"Add State(s) to Queue__jki_lib_state_machine.vi"("State(s) in (\"\")"=w451, "State(s) at Back (\"\")"="Data: Save Controls\nData: Cleanup\nExit") -> ("States Out"=w449:string)  [unwired: 13 in]
        n244 = call <vilib>:"Add State(s) to Queue__jki_lib_state_machine.vi"("State(s) in Front (\"\")"=w449, "State(s) in (\"\")"=w458) -> ("States Out"=w457:string)  [unwired: 13 in]
      }
      frame "Macro: Output" {
        n245 = case shown="False" "I'm Finished Taking Data!" {
          tunnel: [w473 _] -> w462
          frame False {
            n246 = local read "KH Addresses"() -> (w469:refnum<visa-resource-name>[])
            n247 = Empty Array?(array=w469) -> (empty?=w468:bool)
            n248 = Select(t="", s=w468, f="UI: SR Disable\nKH: set KH 0\nKH: set KH 1\nKH: set KH 2" ("State(s) in Front (\"\")")) -> (s? t:f=w470:string)
            n249 = call <vilib>:"Add State(s) to Queue__jki_lib_state_machine.vi"("State(s) in Front (\"\")"="Macro: Initialize Metadata" ("State(s) in Front (\"\")"), "State(s) in (\"\")"=w470, "State(s) at Back (\"\")"="Macro: Write Metadata" ("State(s) in Front (\"\")")) -> ("States Out"=w473:string)  [unwired: 12 in]
          }
          frame True {
          }
        }
        n250 = call <vilib>:"Add State(s) to Queue__jki_lib_state_machine.vi"("State(s) in Front (\"\")"=w462, "State(s) in (\"\")"=w465, "State(s) at Back (\"\")"="PGSQL: Write" ("State(s) in Front (\"\")")) -> ("States Out"=w464:string)  [unwired: 12 in]
      }
      frame "Macro: Initialize Metadata" {
        # "Do not put any code in this frame.\n(It is a separator no-op. You can make a copy of this frame to create a new Macro frame)"
        n251 = call <vilib>:"Add State(s) to Queue__jki_lib_state_machine.vi"("State(s) in Front (\"\")"="Metadata: Update Experiment Description\nMetadata: Update Wiring Configuration\nMetadata: Update KH\nMetadata: Build Path\nMetadata: Update Control Experiment Wire\nInstruments: Load Classes\nInstruments: Initialize KH\nInstruments: Initialize Lockin\nInstruments: Initialize Instruments" ("State(s) in Front (\"\")"), "State(s) in (\"\")"=w478) -> ("States Out"=w477:string)  [unwired: 13 in]
      }
      frame "Macro: Write Metadata" {
        # "Do not put any code in this frame.\n(It is a separator no-op. You can make a copy of this frame to create a new Macro frame)"
        n252 = call <vilib>:"Add State(s) to Queue__jki_lib_state_machine.vi"("State(s) in Front (\"\")"="Metadata: Update Comments\nMetadata: Write JSON\nMetadata: Update FGV\n//Macro: Asana" ("State(s) in Front (\"\")"), "State(s) in (\"\")"=w483) -> ("States Out"=w482:string)  [unwired: 13 in]
      }
      frame "Macro: Asana" {
        # "Do not put any code in this frame.\n(It is a separator no-op. You can make a copy of this frame to create a new Macro frame)"
        n253 = call <vilib>:"Add State(s) to Queue__jki_lib_state_machine.vi"("State(s) in Front (\"\")"="Asana: Authenticate\nAsana: Get Teams and Projects" ("State(s) in Front (\"\")"), "State(s) in (\"\")"=w488) -> ("States Out"=w487:string)  [unwired: 13 in]
      }
      frame "---------- Metadata ----------" {
        n254 = call <vilib>:"Add State(s) to Queue__jki_lib_state_machine.vi"("State(s) in (\"\")"=w492) -> ("States Out"=w491:string)  [unwired: 14 in]
      }
      frame "Metadata: Update Experiment Description" {
        n255 = Concatenate Strings("Sample (SAXXXX)", "." ("string"), "Device (YYYYMMDD)") -> (w496:string)
        n256 = Bundle By Name(cluster=w500, "Experiment.Device"=w496, "Experiment.User"="Username", "Experiment.Device Description"="Description", "Experiment.Instrument"="Instrument") -> (w501:T26)
        n257 = call <vilib>:"Add State(s) to Queue__jki_lib_state_machine.vi"("State(s) in (\"\")"=w504) -> ("States Out"=w503:string)  [unwired: 14 in]
      }
      frame "Metadata: Update Wiring Configuration" {
        n258 = local read "Lockin"() -> (w513:T7)
        n259 = local read "non KH"() -> (w507:T10)
        n260 = local read "Lockin"() -> (w511:T7)
        n261 = Unbundle By Name(w507) -> ("Electrodes 2"=w506:string[], "Labels 2"=w505:u16[])
        n262 = Unbundle By Name(w511) -> ("Electrode Config"=w510:T6[])
        n263 = Unbundle By Name(w513) -> ("AI"=w508:u32[], "Electrode"=w509:string[], "Label"=w512:u16[])
        n264 = for {
          tunnel: w505 -> [w522] mode=indexing
          tunnel: [w521] -> w514 mode=indexing
          n265 = property on="Ring" class="Ring (strict)"() -> ("Strings []"=w523:string[])  [unwired: 2 in, 2 out]
          n266 = Index Array(array=w523, index=w522) -> (element=w521:string)
        }
        n267 = for {
          tunnel: w512 -> [w525] mode=indexing
          tunnel: [w524] -> w515 mode=indexing
          n268 = property on="Ring" class="Ring (strict)"() -> ("Strings []"=w526:string[])  [unwired: 2 in, 2 out]
          n269 = Index Array(array=w526, index=w525) -> (element=w524:string)
        }
        n270 = Bundle By Name(cluster=w516, "Wiring Configuration.Lockin Ch"=w508, "Wiring Configuration.KH.Electrodes"=w509, "Wiring Configuration.KH.Labels"=w515, "Wiring Configuration.not KH.Electrodes"=w506, "Wiring Configuration.not KH.Labels"=w514, "Lockin.Electrode Config"=w510) -> (w517:T26)
        n271 = call <vilib>:"Add State(s) to Queue__jki_lib_state_machine.vi"("State(s) in (\"\")"=w520) -> ("States Out"=w519:string)  [unwired: 14 in]
      }
      frame "Metadata: Update KH" {
        n272 = local read "KH All Buttons"() -> (w540:T8)
        n273 = local read "KH"() -> (w542:T5)
        n274 = Unbundle By Name(w542) -> ("KH #"=w529:u16[], "KH Gain"=w539:T3[], "KH Configuration"=w528:T2[], "KH Shunt Resistor"=w536:T4[])
        n275 = call "Initialize KH Array.vi"("KH #"=w529, "Control in"=w539) -> ("Control out"=w541:variant)  [unwired: 9 in]
        n276 = Variant To Data(error in=w533, type=w539, Variant=w541) -> (data=w538:T3[], error out=w532:errorcluster)
        n277 = call "Initialize KH Array.vi"("KH #"=w529, "Control in"=w528) -> ("Control out"=w537:variant)  [unwired: 9 in]
        n278 = Variant To Data(error in=w532, type=w528, Variant=w537) -> (data=w527:T2[], error out=w531:errorcluster)
        n279 = call "Initialize KH Array.vi"("KH #"=w529, "Control in"=w536) -> ("Control out"=w534:variant)  [unwired: 9 in]
        n280 = Variant To Data(error in=w531, type=w536, Variant=w534) -> (data=w535:T4[], error out=w530:errorcluster)
        n281 = Bundle By Name(cluster=w543, "KH.KH #"=w529, "KH.KH Gain"=w538, "KH.KH Configuration"=w527, "KH.KH Shunt Resistor"=w535, "KH All Buttons"=w540) -> (w544:T26)
        n282 = call <vilib>:"Add State(s) to Queue__jki_lib_state_machine.vi"("State(s) in (\"\")"=w546) -> ("States Out"=w545:string)  [unwired: 14 in]
      }
      frame "Metadata: Build Path" {
        n283 = Unbundle By Name(w558) -> ("Experiment.Instrument"=w555:T9, "Experiment.Device"=w554:string)
        n284 = Format Into String(w555) -> (resulting string=w547:string)  [unwired: 3 in, 1 out]
        n285 = Build Path(base path="Default Path", name or relative path=w547) -> (appended path=w556:path)
        n286 = Build Path(base path=w556, name or relative path=w554) -> (appended path=w553:path)
        n287 = call <userlib>:"MGI Create Directory Chain.vi"("Error In"=w552, "File Presence (Auto Detect)"=MGI_Create_Directory_Chain_Behavior_Enum."Path Does Not Contain a File", "Path"=w553) -> ("Error Out"=w551:errorcluster, "Duplicate Path"=w549:path)  [unwired: 7 in]
        "Device Folder" <- w549
        n288 = Bundle By Name(cluster=w558, "Experiment.Device Path"=w549) -> (w557:T26)
        n289 = call <vilib>:"Add State(s) to Queue__jki_lib_state_machine.vi"("State(s) in (\"\")"=w560) -> ("States Out"=w559:string)  [unwired: 14 in]
      }
      frame "Metadata: Update Control Experiment Wire" {
        # "IS Control Experiment Class wire"
        # "Not on Control Experiment Class wire"
        n290 = call-poly <userlib>:"File Exists__ogtk.vi"("file path"="AWS Credentials") -> ("exists"=w563:bool)  [unwired: 6 in, 1 out]
        n291 = First Call?() -> (First Call?: T/F=w564:bool)
        n292 = Not(x=w563) -> (.not. x?=w561:bool)
        n293 = And(x=w561, y=w564) -> (x .and. y?=w562:bool)
        n294 = case shown="True" w562 {
          tunnel: "AWS Credentials" -> [w577 _]
          tunnel: [w577 _] -> w566
          tunnel: "https://docs.aws.amazon.com/cli/latest/userguide/cli-configure-files.html" ("URL") -> [_ w578]
          frame False {
          }
          frame True {
            n295 = call "Display Message to User"() -> ("OK"=w579:bool)  [unwired: 10 in, 1 out]
            n296 = case shown="True" w579 {
              tunnel: w578 -> [_ w580]
              frame False {
              }
              frame True {
                n297 = call-poly <vilib>:"Open URL in Default Browser.vi"("URL"=w580) -> ()  [unwired: 5 in, 2 out]
              }
            }
          }
        }
        n298 = Unbundle By Name(w572) -> ("C.E."=w570:refnum<class "Control Experiment SM.lvclass">, "Experiment"=w574:T21, "Wiring Configuration"=w573:T22)
        n299 = Bundle By Name(cluster=w570, "Experiment"=w574, "Wiring Configuration"=w573, "AWS Credentials"=w566) -> (w568:refnum<class "Control Experiment SM.lvclass">)
        n300 = Bundle By Name(cluster=w572, "C.E."=w568) -> (w571:T26)
        n301 = call <vilib>:"Add State(s) to Queue__jki_lib_state_machine.vi"("State(s) in (\"\")"=w576) -> ("States Out"=w575:string)  [unwired: 14 in]
      }
      frame "Metadata: Update Comments" {
        # "error 63 occurs when\nthe lockin isn't running\nI think we can clear here?"
        n302 = Unbundle By Name(w591) -> ("C.E."=w587:refnum<class "Control Experiment SM.lvclass">)
        n303 = call "Generate Comments.vi"("error in (no error)"=w582, "Control Experiment"=w587) -> ("error out"=w584:errorcluster, "Control Experiment out"=w586:refnum<class "Control Experiment SM.lvclass">)  [unwired: 6 in, 1 out]
        n304 = call <vilib>:"Clear Errors.vi"("error in (no error)"=w584, "specific error code to clear (0: all)"=63) -> ("error out"=w583:errorcluster)  [unwired: 4 in, 1 out]
        n305 = call "Read Comments.vi"("error in (no error)"=w583, "Control Experiment in"=w586) -> ("error out"=w581:errorcluster, "Comments"=→"Comments":string, "Control Experiment out"=w588:refnum<class "Control Experiment SM.lvclass">)  [unwired: 7 in]
        n306 = Bundle By Name(cluster=w591, "C.E."=w588) -> (w590:T26)
        n307 = call <vilib>:"Add State(s) to Queue__jki_lib_state_machine.vi"("State(s) in (\"\")"=w593) -> ("States Out"=w592:string)  [unwired: 14 in]
      }
      frame "Metadata: Update FGV" {
        n308 = Unbundle By Name(w598) -> ("C.E."=w595:refnum<class "Control Experiment SM.lvclass">)
        n309 = call "Control Experiment FGV.vi"("Function"=enum16{"read", "write"}."write", "error in (no error)"=w594, "Control Experiment.lvclass"=w595) -> ("error out"=w596:errorcluster)  [unwired: 7 in, 1 out]
        n310 = call <vilib>:"Add State(s) to Queue__jki_lib_state_machine.vi"("State(s) in (\"\")"=w600) -> ("States Out"=w599:string)  [unwired: 14 in]
      }
      frame "Metadata: Write JSON" {
        w611 = T31 {"Device"={"Device"="", "User"="", "Time"="", "Computer Name"=""}, "Wiring"={"Lockin Ch"=[], "KH Electrodes"=[], "KH Labels"=[], "Other Electrodes"=[], "Other Labels"=[]}}  # Control Experiment JSON
        n311 = Unbundle By Name(w603) -> ("C.E."=w612:refnum<class "Control Experiment SM.lvclass">, "Experiment.Device"=w627:string, "Experiment.User"=w626:string)
        n312 = Unbundle By Name(w603) -> ("Lockin.AI"=w625:u32[], "Wiring Configuration.KH.Electrodes"=w624:string[], "Wiring Configuration.KH.Labels"=w623:string[], "Wiring Configuration.KH.Electrodes"=w621:string[], "Wiring Configuration.KH.Labels"=w620:string[])
        n313 = call "Get Date Time ISO.vi"("error in (no error)"=w619) -> ("error out"=w616:errorcluster, "ISO 8601 date-time string"=w617:string)  [unwired: 8 in, 1 out]
        n314 = call "GetLocalComputerName.vi"("error in (no error)"=w616) -> ("error out"=w618:errorcluster, "Name"=w622:string)  [unwired: 8 in, 1 out]
        n315 = Bundle By Name(cluster=w611, "Device.Device"=w627, "Device.User"=w626, "Device.Time"=w617, "Device.Computer Name"=w622) -> (w610:T31)
        n316 = Bundle By Name(cluster=w610, "Wiring.Lockin Ch"=w625, "Wiring.KH Electrodes"=w624, "Wiring.KH Labels"=w623, "Wiring.Other Electrodes"=w621, "Wiring.Other Labels"=w620) -> (w609:T31)
        n317 = call <vilib>:"Flatten To JSON String.vi"("Enums As String (F)"=TRUE, "error in (no error)"=w618, "Variant"=w609) -> ("error out"=w614:errorcluster, "JSON String"=→"JSON String":string)  [unwired: 7 in]
        n318 = call "Write Experiment Folder.vi"("error in (no error)"=w614, "Experiment Folder"="device", "Control Experiment in"=w612) -> ("error out"=w613:errorcluster, "Control Experiment out"=w615:refnum<class "Control Experiment SM.lvclass">)  [unwired: 7 in]
        n319 = call "Save JSON File.vi"("error in (no error)"=w613, "Data"=w609, "Control Experiment in"=w615) -> ("error out"=w605:errorcluster, "JSON String"=w606:string, "Control Experiment out"=w607:refnum<class "Control Experiment SM.lvclass">)  [unwired: 6 in]
        n320 = call "Write Device Description JSON.vi"("error in (no error)"=w605, "Device Description JSON"=w606, "Control Experiment in"=w607) -> ("error out"=w604:errorcluster, "Control Experiment out"=w601:refnum<class "Control Experiment SM.lvclass">)  [unwired: 7 in]
        n321 = Bundle By Name(cluster=w603, "C.E."=w601) -> (w602:T26)
        n322 = call <vilib>:"Add State(s) to Queue__jki_lib_state_machine.vi"("State(s) in (\"\")"=w631) -> ("States Out"=w630:string)  [unwired: 14 in]
      }
      frame "---------- KH ----------" {
        n323 = call <vilib>:"Add State(s) to Queue__jki_lib_state_machine.vi"("State(s) in (\"\")"=w635) -> ("States Out"=w634:string)  [unwired: 14 in]
      }
      frame "KH: set KH 0" {
        # "initialize the Channel Settings array"
        # "remove duplicates"
        n324 = local read "KH Addresses"() -> (w648:refnum<visa-resource-name>[])
        n325 = call-poly <userlib>:"Remove Duplicates from 1D Array__ogtk.vi"("Input Array"=w648) -> ("Output Array"=w649:variant[])  [unwired: 1 out]
        n326 = Variant To Data(error in=w647, type=w648, Variant=w649) -> (data=w640:refnum<visa-resource-name>[], error out=w639:errorcluster)
        n327 = local write "KH Addresses"(w640) -> ()
        n328 = Initialize Array(T15 {"Channel"=enum."Channel 1", "Gain"=enum."10x", "Bandwidth Filter"=enum."ON", "Shunt Resistor"=enum."50 Ohms", "Coupling"=enum."DC", "Input Config"=enum."Differential"} ("Channel Settings"), 8 ("dimension size")) -> (w642:T15[])
        n329 = Bundle(w642) -> (w641:cluster{T15[]})  [unwired: 1 in]
        n330 = Array Size(array=w640) -> (size(s)=w645:i32)
        n331 = for {
          tunnel: w640 -> [_] mode=indexing
          tunnel: [w657] -> w636 mode=concatenating
          tunnel: w639 -> [w656]
          tunnel: [w655] -> w638
          i -> [w659]
          n332 = call "Number to Letter.vi"("Number"=w659) -> ("Letter"=w658:string)
          n333 = for {
            N: 8 -> [_]
            tunnel: w658 -> [w664]
            tunnel: [w663] -> w657 mode=indexing
            tunnel: w656 -> [w662]
            tunnel: [w661] -> w655
            i -> [w666]
            n334 = Increment(x=w666) -> (x+1=w660:i32)
            n335 = Format Into String(format string="%s %d", error in=w662, w664, w660) -> (resulting string=w663:string, error out=w661:errorcluster)  [unwired: 1 in]
          }
        }
        n336 = Initialize Array(w641, w645) -> (w646:cluster{T15[]}[])
        n337 = Bundle By Name(cluster=w651, "Channel Settings"=w646) -> (w650:T26)
        n338 = property on="Ring" class="Ring (strict)"(error in=w638, "Strings []"=w636) -> (error out=w637:errorcluster)  [unwired: 1 in, 1 out]
        n339 = call <vilib>:"Add State(s) to Queue__jki_lib_state_machine.vi"("State(s) in (\"\")"=w653) -> ("States Out"=w652:string)  [unwired: 14 in]
      }
      frame "KH: set KH 1" {
        n340 = Unbundle By Name(w678) -> ("Channel Settings"=w667:cluster{"Channel Setting":T23}[], "KH.KH #"=w680:u16[], "KH.KH Gain"=w683:T3[], "Lockin.Electrode Config"=w681:T6[], "KH.KH Shunt Resistor"=w682:T4[], "KH All Buttons"=w679:T8)
        n341 = local read "Bandwidth Filter"() -> (w668:bool)
        n342 = local read "DC Coupled"() -> (w669:bool)
        n343 = for {
          tunnel: w681 -> [w708] mode=indexing
          tunnel: w683 -> [w707] mode=indexing
          tunnel: w682 -> [w706] mode=indexing
          tunnel: w680 -> [w702] mode=indexing
          tunnel: [w711] -> w674 mode=indexing
          tunnel: w679 -> [w710]
          tunnel: [w709] -> w672 mode=indexing
          tunnel: [w705] -> w673 mode=indexing
          shift-right: [w698] -> w676
          shift-left: w667 -> [w699]
          tunnel: w669 -> [w694]
          tunnel: w668 -> [w689]
          n344 = property on="Ring" class="Ring (strict)"() -> ("Strings []"=w704:string[])  [unwired: 2 in, 2 out]
          n345 = case shown="\"No Selection\", Default" w710 {
            tunnel: w708 -> [w730 _ _]
            tunnel: [w735 Input_Configuration-Enum."Ground" ("Input Config") Input_Configuration-Enum."Differential" ("Input Config")] -> w705
            tunnel: w707 -> [w734 w753 w756]
            tunnel: [w733 w753 w756] -> w709
            tunnel: w706 -> [w732 _ _]
            tunnel: [w731 Shunt-Enum."Open" ("Shunt Resistor") w754] -> w711
            frame "No Selection", Default {
              n346 = case shown="\"Voltage (SE)\"" w730 {
                tunnel: [Input_Configuration-Enum."Ground" ("Input Config") Input_Configuration-Enum."Differential" ("Input Config") Input_Configuration-Enum."SE+ (-gnd)" ("Input Config") Input_Configuration-Enum."Differential" ("Input Config") Input_Configuration-Enum."Differential" ("Input Config")] -> w735
                tunnel: [Shunt-Enum."Open" ("Shunt Resistor") w739 Shunt-Enum."Open" ("Shunt Resistor") Shunt-Enum."Open" ("Shunt Resistor") Shunt-Enum."50k Ohms" ("Shunt Resistor")] -> w731
                tunnel: w734 -> [w736 w740 w743 w747 w749]
                tunnel: [w736 w740 w743 w747 w749] -> w733
                tunnel: w732 -> [_ w739 _ _ _]
                frame "Ground", Default {
                }
                frame "Current" {
                }
                frame "Voltage (SE)" {
                }
                frame "Voltage (Diff)" {
                }
                frame "Gate" {
                }
              }
            }
            frame "All Ground" {
            }
            frame "All Differential" {
              n347 = local read "Defualt Shunt Resistor"() -> (w754:T4)
            }
          }
          n348 = To Long Integer(number=w702) -> (32bit integer=w703:i32)
          n349 = Index Array(array=w704, index=w703) -> (element=w701:string)
          n350 = Select(t=Coupling-Enum."DC" ("Coupling"), s=w694, f=Coupling-Enum."AC" ("Coupling")) -> (s? t:f=w691:T18)
          n351 = Scan From String(format string="%s %d", input string=w701) -> (error out=w695:errorcluster, output 1=w697:string, output 2=w696:i32)  [unwired: 4 in, 2 out]
          n352 = Select(t=Filter-Enum."ON" ("Bandwidth Filter"), s=w689, f=Filter-Enum."OFF" ("Bandwidth Filter")) -> (s? t:f=w687:T17)
          n353 = case shown="No Error" w695 {
            tunnel: w711 -> [w728 _]
            tunnel: w709 -> [w727 _]
            tunnel: w705 -> [w726 _]
            tunnel: w699 -> [w718 w729]
            tunnel: [w717 w729] -> w698
            tunnel: w697 -> [w716 _]
            tunnel: w696 -> [w715 _]
            tunnel: w691 -> [w713 _]
            tunnel: w687 -> [w712 _]
            frame No Error {
              n354 = Decrement(x=w715) -> (x-1=w714:i32)
              n355 = call "Letter to Number.vi"("Letter"=w716) -> ("Number"=w719:i32)
              n356 = Index Array(array=w718, index=w719) -> (element=w724:cluster{"Channel Setting":T23})
              n357 = Unbundle(w724) -> ("Channel Setting"=w723:T23)
              n358 = Index Array(array=w723, index=w714) -> (element=w722:T15)
              n359 = Bundle By Name(cluster=w722, "Channel"=w714, "Gain"=w727, "Input Config"=w726, "Shunt Resistor"=w728, "Coupling"=w713, "Bandwidth Filter"=w712) -> (w721:T15)
              n360 = Replace Array Subset(array=w723, new element=w721, index=w714) -> (w725:T23)
              n361 = Bundle("Channel Setting"=w725) -> (w720:cluster{"Channel Setting":T23})  [unwired: 1 in]
              n362 = Replace Array Subset(array=w718, new element=w720, index=w719) -> (w717:cluster{"Channel Setting":T23}[])
            }
            frame Error {
            }
          }
        }
        n363 = local write "KH All Buttons"(T8."No Selection" ("KH All Buttons")) -> ()
        n364 = Bundle By Name(cluster=w678, "Channel Settings"=w676, "KH.KH Gain"=w672, "KH.KH Configuration"=w673, "KH.KH Shunt Resistor"=w674) -> (w684:T26)
        n365 = local read "KH"() -> (w675:T5)
        n366 = Bundle By Name(cluster=w675, "KH Gain"=w672, "KH Configuration"=w673, "KH Shunt Resistor"=w674) -> (w671:T5)
        n367 = local write "KH"(w671) -> ()
        n368 = call <vilib>:"Add State(s) to Queue__jki_lib_state_machine.vi"("State(s) in (\"\")"=w686) -> ("States Out"=w685:string)  [unwired: 14 in]
      }
      frame "KH: set KH 2" {
        n369 = Unbundle By Name(w764) -> ("Channel Settings"=w769:cluster{"Channel Setting":T23}[])
        n370 = Unbundle By Name(w764) -> ("C.E."=w761:refnum<class "Control Experiment SM.lvclass">)
        n371 = Unbundle By Name(w761) -> ("KH7008"=w760:refnum<class "Instrument.KH7008.lvclass">[])
        n372 = for {
          tunnel: w759 -> [w784]
          tunnel: [w776] -> w757
          tunnel: w769 -> [w783] mode=indexing
          tunnel: w760 -> [w782] mode=indexing
          tunnel: [w775] -> w765 mode=concatenating
          tunnel: [w774] -> w758 mode=indexing
          n373 = Unbundle(w783) -> ("Channel Setting"=w779:T23)
          n374 = call <userlib>:"Write Channel Setting.vi"("error in (no error)"=w784, "Channel Setting"=w779, "KH7008 in"=w782) -> ("error out"=w780:errorcluster, "KH7008 out"=w781:refnum<class "Instrument.KH7008.lvclass">)  [unwired: 7 in]
          n375 = call <userlib>:"KH Control.vi"("error in"=w780, "KH7008.lvclass"=w781) -> ("error out"=w778:errorcluster, "KH7008.lvclass out"=w777:refnum<class "Instrument.KH7008.lvclass">)  [unwired: 8 in]
          n376 = call <userlib>:"Read Gain.vi"("error in (no error)"=w778, "KH7008 in"=w777) -> ("error out"=w776:errorcluster, "Gain"=w775:dbl[], "KH7008 out"=w774:refnum<class "Instrument.KH7008.lvclass">)  [unwired: 7 in]
        }
        n377 = local read "Gain"() -> (w766:dbl[])
        n378 = Bundle By Name(cluster=w761, "KH7008"=w758) -> (w763:refnum<class "Control Experiment SM.lvclass">)
        n379 = call "Multiply Gains.vi"("Other Gain"=w766, "Gain"=w765) -> ("Gain x Other Gain"=w768:dbl[])
        n380 = Unbundle By Name(w763) -> ("Lockin"=w762:refnum<class "Instrument.Lockin.lvclass">)
        n381 = call <userlib>:"setInputGain.vi"("error in (no error)"=w757, "InputGain"=w768, "Instrument.Lockin in"=w762) -> ("error out"=w767:errorcluster)  [unwired: 7 in, 1 out]
        n382 = Bundle By Name(cluster=w764, "C.E."=w763) -> (w771:T26)
        n383 = call <vilib>:"Clear Errors.vi"("error in (no error)"=w767) -> ("error out"=w770:errorcluster)  [unwired: 5 in, 1 out]
        n384 = call <vilib>:"Add State(s) to Queue__jki_lib_state_machine.vi"("State(s) in (\"\")"=w773) -> ("States Out"=w772:string)  [unwired: 14 in]
      }
      frame "---------- Instruments ----------" {
        n385 = call <vilib>:"Add State(s) to Queue__jki_lib_state_machine.vi"("State(s) in (\"\")"=w788) -> ("States Out"=w787:string)  [unwired: 14 in]
      }
      frame "Instruments: Load Classes" {
        n386 = Unbundle By Name(w794) -> ("C.E."=w792:refnum<class "Control Experiment SM.lvclass">)
        n387 = call "Load Instrument Classes.vi"("error in (no error)"=w789, "Control Experiment.lvclass"=w792) -> ("error out"=w790:errorcluster, "Control Experiment out"=w791:refnum<class "Control Experiment SM.lvclass">)  [unwired: 8 in]
        n388 = Bundle By Name(cluster=w794, "C.E."=w791) -> (w793:T26)
        n389 = call <vilib>:"Add State(s) to Queue__jki_lib_state_machine.vi"("State(s) in (\"\")"=w796) -> ("States Out"=w795:string)  [unwired: 14 in]
      }
      frame "Instruments: Initialize KH" {
        n390 = Unbundle By Name(w800) -> ("C.E."=w801:refnum<class "Control Experiment SM.lvclass">)
        n391 = Unbundle By Name(w801) -> ("KH7008"=w803:refnum<class "Instrument.KH7008.lvclass">[])
        n392 = for {
          tunnel: w803 -> [w809]
          tunnel: [w813] -> w797 mode=indexing
          tunnel: w805 -> [w812]
          tunnel: [w811] -> w804
          tunnel: "KH Addresses" -> [w810] mode=indexing
          n393 = Index Array(array=w809) -> (element=w808:refnum<class "Instrument.KH7008.lvclass">)  [unwired: 1 in]
          n394 = call-dynamic "Open.vi"("error in (no error)"=w812, "Address"=w810, "Instrument.KH7008 in"=w808) -> ("error out"=w811:errorcluster, "Instrument.KH7008 out"=w813:refnum<class "Instrument.KH7008.lvclass">)  [unwired: 7 in]
        }
        n395 = Bundle By Name(cluster=w801, "KH7008"=w797) -> (w798:refnum<class "Control Experiment SM.lvclass">)
        n396 = Bundle By Name(cluster=w800, "C.E."=w798) -> (w799:T26)
        n397 = call <vilib>:"Add State(s) to Queue__jki_lib_state_machine.vi"("State(s) in (\"\")"=w807) -> ("States Out"=w806:string)  [unwired: 14 in]
      }
      frame "Instruments: Initialize Lockin" {
        n398 = Unbundle By Name(w820) -> ("C.E."=w816:refnum<class "Control Experiment SM.lvclass">)
        n399 = Unbundle By Name(w816) -> ("Lockin"=w817:refnum<class "Instrument.Lockin.lvclass">)
        n400 = call-dynamic "Open.vi"("error in (no error)"=w821, "Address"="Lockin Address", "Instrument.Lockin in"=w817) -> ("error out"=w818:errorcluster, "Instrument.Lockin out"=w815:refnum<class "Instrument.Lockin.lvclass">)  [unwired: 7 in]
        n401 = Bundle By Name(cluster=w816, "Lockin"=w815) -> (w814:refnum<class "Control Experiment SM.lvclass">)
        n402 = Bundle By Name(cluster=w820, "C.E."=w814) -> (w819:T26)
        n403 = call <vilib>:"Add State(s) to Queue__jki_lib_state_machine.vi"("State(s) in (\"\")"=w824) -> ("States Out"=w823:string)  [unwired: 14 in]
      }
      frame "Instruments: Initialize Instruments" {
        n404 = Unbundle By Name(w831) -> ("C.E."=w830:refnum<class "Control Experiment SM.lvclass">)
        n405 = Unbundle By Name(w830) -> ("Capacitance Bridge"=w836:refnum<class "Instrument.CBridge.lvclass">, "Strain Cell"=w826:refnum<class "Instrument.Strain.lvclass">)
        n406 = call-dynamic "Open.vi"("error in (no error)"=w832, "Address"="Capacitance Bridge Address", "Instrument in"=w836) -> ("error out"=w835:errorcluster, "Instrument out"=w829:refnum<class "Instrument.CBridge.lvclass">)  [unwired: 7 in]
        n407 = call-dynamic "Open.vi"("error in (no error)"=w835, "Address"="Strain Cell Address", "Instrument in"=w826) -> ("error out"=w825:errorcluster, "Instrument out"=w827:refnum<class "Instrument.Strain.lvclass">)  [unwired: 7 in]
        n408 = Bundle By Name(cluster=w830, "Capacitance Bridge"=w829, "Strain Cell"=w827) -> (w828:refnum<class "Control Experiment SM.lvclass">)
        n409 = Bundle By Name(cluster=w831, "C.E."=w828) -> (w837:T26)
        n410 = call <vilib>:"Add State(s) to Queue__jki_lib_state_machine.vi"("State(s) in (\"\")"=w839) -> ("States Out"=w838:string)  [unwired: 14 in]
      }
      frame "---------- Asana ----------" {
        n411 = call <vilib>:"Add State(s) to Queue__jki_lib_state_machine.vi"("State(s) in (\"\")"=w843) -> ("States Out"=w842:string)  [unwired: 14 in]
      }
      frame "Asana: Initialize Authentication Info" {
        n412 = Bundle By Name(cluster=w845, "Asana.Authentication Info.Client ID"="1150712142949183" ("Client ID"), "Asana.Authentication Info.Client Secret"="530770942aed47201cd52aeb331bdd57" ("Client Secret"), "Asana.Authentication Info.Redirect URI"="https://www.google.com/" ("Redirect URI")) -> (w844:T26)
        n413 = call <vilib>:"Add State(s) to Queue__jki_lib_state_machine.vi"("State(s) in (\"\")"=w851) -> ("States Out"=w850:string)  [unwired: 14 in]
      }
      frame "Asana: Authenticate" {
        n414 = Unbundle By Name(w853) -> ("Asana.Time Stamp"=w867:timestamp, "Asana.Refresh Token"=w854:string, "Asana.Authentication Info"=w857:T32)
        n415 = Get Date/Time In Seconds() -> (seconds since 1Jan1904=w866:timestamp)
        n416 = Subtract(x=w867, y=w866) -> (x-y=w865:dbl)
        n417 = Less?(x=w865, y=3600.0) -> (x < y?=w858:bool)
        n418 = Select(t=w854, s=w858, f="" ("t")) -> (s? t:f=w856:string)
        n419 = call <userlib>:"Asana Authentication.vi"("error in (no error)"=w852, "Authentication Info"=w857, "Refresh Token In"=w856) -> ("error out"=w861:errorcluster, "Authentication Header"=w860:T25[], "Refresh Token Out"=w859:string)  [unwired: 5 in, 1 out]
        n420 = case shown="No Error" w861 {
          selector: w861 -> [w871 _]
          tunnel: w860 -> [w872 _]
          tunnel: w859 -> [w870 _]
          tunnel: w853 -> [w875 w877]
          tunnel: [w873 w877] -> w863
          tunnel: [w871 errorcluster {"status"=FALSE, "code"=0, "source"=""} ("error in (no error)")] -> w862
          frame No Error {
            n421 = Get Date/Time In Seconds() -> (seconds since 1Jan1904=w874:timestamp)
            n422 = Bundle By Name(cluster=w875, "Asana.Refresh Token"=w870, "Asana.Authentication Header"=w872, "Asana.Time Stamp"=w874) -> (w873:T26)
            "Refresh Token Out" <- w870
          }
          frame Error {
          }
        }
        n423 = call <vilib>:"Add State(s) to Queue__jki_lib_state_machine.vi"("State(s) in (\"\")"=w869) -> ("States Out"=w868:string)  [unwired: 14 in]
      }
      frame "Asana: Get Teams and Projects" {
        # "task"
        # "project"
        # "team"
        n424 = Unbundle By Name(w885) -> ("Asana.Authentication Header"=w881:T25[])
        n425 = Unbundle By Name(w885) -> ("Experiment.Device"=w878:string)
        n426 = call <userlib>:"Get Teams.vi"("Authorization"=w881, "error in (no error)"=w898) -> ("error out"=w897:errorcluster, "Teams Out"=w887:T33)  [unwired: 8 in]
        n427 = Format Into String(error in=w897, T19."Samples" ("Team")) -> (resulting string=w896:string, error out=w895:errorcluster)  [unwired: 2 in]
        n428 = call "Asana Dictionary Get Value.vi"("error in (no error)"=w895, "Key"=w896, "Data"=w887) -> ("error out"=w892:errorcluster, "Value"=w894:string)  [unwired: 7 in]
        n429 = call <userlib>:"Get Projects.vi"("Authorization"=w881, "error in (no error)"=w892, "Team GID"=w894) -> ("error out"=w891:errorcluster, "Projects Out"=w889:T33)  [unwired: 7 in]
        n430 = call "Asana Dictionary Get Value.vi"("error in (no error)"=w891, "Key"="Devices" ("element"), "Data"=w889) -> ("error out"=w890:errorcluster, "Value"=w879:string)  [unwired: 7 in]
        n431 = call <userlib>:"Get Tasks.vi"("Authorization"=w881, "error in (no error)"=w890, "Project GID"=w879) -> ("error out"=w886:errorcluster, "data"=w888:T34)  [unwired: 7 in]
        n432 = call "Asana Dictionary Tasks Get Value.vi"("error in (no error)"=w886, "Key"=w878, "data"=w888) -> ("error out"=w883:errorcluster, "Value"=w884:string)  [unwired: 7 in]
        n433 = case shown="\"\"" w884 {
          tunnel: w883 -> [w901 w906]
          tunnel: [w901 w905] -> w882
          tunnel: w881 -> [_ w904]
          tunnel: w879 -> [_ w903]
          tunnel: w878 -> [_ w902]
          frame Default {
          }
          frame "" {
            # "empty means\ntask doesn't\nexist"
            n434 = case shown="Default" w902 {
              selector: w902 -> [_ w908]
              tunnel: w906 -> [w907 w912]
              tunnel: [w907 w911] -> w905
              tunnel: w904 -> [_ w910]
              tunnel: w903 -> [_ w909]
              frame "" {
              }
              frame Default {
                n435 = call <userlib>:"Create Task.vi"("Authorization"=w910, "error in (no error)"=w912, "Name"=w908, "Project GID"=w909) -> ("error out"=w911:errorcluster)  [unwired: 6 in, 1 out]
              }
            }
          }
        }
        n436 = call <vilib>:"Add State(s) to Queue__jki_lib_state_machine.vi"("State(s) in (\"\")"=w900) -> ("States Out"=w899:string)  [unwired: 14 in]
      }
      frame "---------- Experiment VI ----------" {
        n437 = call <vilib>:"Add State(s) to Queue__jki_lib_state_machine.vi"("State(s) in (\"\")"=w916) -> ("States Out"=w915:string)  [unwired: 14 in]
      }
      frame "Experiment VI: Populate VI Ring" {
        n438 = call <userlib>:"Current VIs Parent Directory__ogtk.vi"() -> ("Parent Directory (+ Relative)"=w933:path)  [unwired: 5 in]
        n439 = call <userlib>:"String to 1D Array__ogtk.vi"("delimiter (Tab)"="\n", "string"="----Sweep Control----\nSweep Control.vi\nContinuous B Sweep.vi") -> ("Array of Strings"=w919:string[])  [unwired: 9 in]
        n440 = call <userlib>:"String to 1D Array__ogtk.vi"("delimiter (Tab)"="\n", "string"="----Transport----\nIV.vi\nIV_Sweep.vi\nLockin_time.vi\nLockin_Vsg.vi\nLockin_sweep.vi\nLockin_AIWFM_time.vi\nTHz_TimeDelay.vi\nSweep_AIWFM_time.vi") -> ("Array of Strings"=w918:string[])  [unwired: 9 in]
        n441 = Strip Path(path=w933) -> (stripped path=w930:path)  [unwired: 1 out]
        n442 = Build Path(base path=w930, name or relative path="SweepControl") -> (appended path=w929:path)
        n443 = Build Path(base path=w930, name or relative path="Transport") -> (appended path=w925:path)
        n444 = for {
          tunnel: w929 -> [w943]
          tunnel: w919 -> [w942] mode=indexing
          tunnel: [w941] -> w922 mode=indexing
          n445 = Build Path(base path=w943, name or relative path=w942) -> (appended path=w941:path)
        }
        n446 = for {
          tunnel: w925 -> [w940]
          tunnel: w918 -> [w939] mode=indexing
          tunnel: [w938] -> w921 mode=indexing
          n447 = Build Path(base path=w940, name or relative path=w939) -> (appended path=w938:path)
        }
        n448 = Build Array (concatenate)(w922, w921) -> (w920:path[])
        n449 = Build Array (concatenate)(w919, w918) -> (w917:string[])
        n450 = Bundle By Name(cluster=w924, "VI paths"=w920) -> (w923:T26)
        n451 = property on="Ring" class="Ring (strict)"("Strings []"=w917) -> ()  [unwired: 2 in, 2 out]
        n452 = call <vilib>:"Add State(s) to Queue__jki_lib_state_machine.vi"("State(s) in (\"\")"=w937) -> ("States Out"=w936:string)  [unwired: 14 in]
      }
      frame "Experiment VI: Open VI" {
        n453 = Unbundle By Name(w949) -> ("VI paths"=w948:path[])
        n454 = Index Array(array=w948, index="Ring") -> (element=w946:path)
        n455 = call "Open Experiment VI.vi"("error in (no error)"=w945, "Path"=w946) -> ("error out"=w944:errorcluster)  [unwired: 9 in]
        n456 = call <vilib>:"Add State(s) to Queue__jki_lib_state_machine.vi"("State(s) in (\"\")"=w951) -> ("States Out"=w950:string)  [unwired: 14 in]
      }
      frame "Experiment VI: Open Lockin" {
        n457 = call "Open Lockin.vi"("error in (no error)"=w953) -> ("error out"=w952:errorcluster)  [unwired: 10 in]
        n458 = call <vilib>:"Add State(s) to Queue__jki_lib_state_machine.vi"("State(s) in (\"\")"=w956) -> ("States Out"=w955:string)  [unwired: 14 in]
      }
      frame "---------- PGSQL ----------" {
        n459 = call <vilib>:"Add State(s) to Queue__jki_lib_state_machine.vi"("State(s) in (\"\")"=w960) -> ("States Out"=w959:string)  [unwired: 14 in]
      }
      frame "PGSQL: Start Logger" {
        n460 = Unbundle By Name(w962) -> ("Logger"=w967:refnum<class "Logger.PGSQL.lvclass">)
        n461 = call <vilib>:"Create.vi"("error in (no error)"=w964, "SMO"=w967) -> ("error out"=w966:errorcluster, "SMO out"=w968:refnum<class "Logger.PGSQL.lvclass">)  [unwired: 7 in, 1 out]
        n462 = call <vilib>:"Start.vi"("error in (no error)"=w966, "SMO"=w968) -> ("error out"=w963:errorcluster, "SMO out"=w965:refnum<class "Logger.PGSQL.lvclass">)  [unwired: 8 in]
        n463 = Bundle By Name(cluster=w962, "Logger"=w965) -> (w961:T26)
        n464 = call <vilib>:"Add State(s) to Queue__jki_lib_state_machine.vi"("State(s) in (\"\")"=w970) -> ("States Out"=w969:string)  [unwired: 14 in]
      }
      frame "PGSQL: Write" {
        w982 = "" ("f")
        n465 = Unbundle By Name(w986) -> ("Logger"=w980:refnum<class "Logger.PGSQL.lvclass">, "Experiment.Instrument"=w971:T9, "Experiment.Device"=w985:string, "Experiment.User"=w984:string)
        n466 = local read "I'm Finished Taking Data!"() -> (w983:bool)
        n467 = Not(x=w983) -> (.not. x?=w981:bool)
        n468 = call "Device and User PGSQL Paths.vi"("instrument"=w971) -> ("User Path"=w973:string, "Device Path"=w979:string)  [unwired: 5 in]
        n469 = Select(t=w985, s=w981, f=w982) -> (s? t:f=w978:string)
        n470 = Select(t=w984, s=w981, f=w982) -> (s? t:f=w972:string)
        n471 = call <userlib>:"Logger.PGSQL.WriteVariable.vi"("error in (no error)"=w976, "Data"=w978, "Address"=w979, "Logger"=w980) -> ("error out"=w975:errorcluster, "Logger out"=w977:refnum<class "Logger.PGSQL.lvclass">)  [unwired: 6 in]
        n472 = call <userlib>:"Logger.PGSQL.WriteVariable.vi"("error in (no error)"=w975, "Data"=w972, "Address"=w973, "Logger"=w977) -> ("error out"=w974:errorcluster)  [unwired: 6 in, 1 out]
        n473 = call <vilib>:"Add State(s) to Queue__jki_lib_state_machine.vi"("State(s) in (\"\")"=w988) -> ("States Out"=w987:string)  [unwired: 14 in]
      }
      frame "---------- Pickering ----------" {
        n474 = call <vilib>:"Add State(s) to Queue__jki_lib_state_machine.vi"("State(s) in (\"\")"=w992) -> ("States Out"=w991:string)  [unwired: 14 in]
      }
    }
  }
  n475 = Unbundle By Name(w2) -> ("C.E."=→"Control Experiment":refnum<class "Control Experiment SM.lvclass">)
